vi "CameraOption Disp.vi"() -> ()   [LabVIEW 2015]
uses:
  global.vi
panel:
  in  "タブ制御器":enum32{"I/O", "Partition"}(tab)
  in  "I/O PortSetting":T1={"ExternalOut2"=13, "ExternalIn2"=6, "ExternalOut1"=0, "ExternalIn1"=0, "ExternalOut3"=13, "ExternalOut4"=13, "ExternalIn3"=6} {"ExternalIn3" items=["TRIG POS "=8, "TRIG NEG "=9]; "ExternalOut4" items=["TRIG POS"=5, "TRIG NEG"=6, ""=11, ""=12]; "ExternalOut3" items=["SYNC POS"=1, "SYNC NEG"=2, "EXPOSE POS"=13, "EXPOSE NEG"=14, "REC POS"=3, "REC NEG"=4, "TRIG POS"=5, "TRIG NEG"=6, "READY POS"=7, "READY NEG"=8, "IRIG RESET POS"=9, "IRIG RESET NEG"=10]; "ExternalIn1" items=["OFF"=1, "CAMSYNC_POS"=2, "CAMSYNC_NEG"=3, "OTHERSSYNC_POS"=4, "OTHERSSYNC_NEG"=5]; "ExternalOut1" items=["SYNC POS"=1, "SYNC NEG"=2, "EXPOSE POS"=13, "EXPOSE NEG"=14, "REC POS"=3, "REC NEG"=4, "TRIG POS"=5, "TRIG NEG"=6, "READY POS"=7, "READY NEG"=8, "IRIG RESET POS"=9, "IRIG RESET NEG"=10]; "ExternalIn2" items=["EVENT POS"=6, "EVENT NEG"=7, "TRIG POS "=8, "TRIG NEG "=9, "READY POS "=10, "READY NEG"=11]; "ExternalOut2" items=["SYNC POS"=1, "SYNC NEG"=2, "EXPOSE POS"=13, "EXPOSE NEG"=14, "REC POS"=3, "REC NEG"=4, "TRIG POS"=5, "TRIG NEG"=6, "READY POS"=7, "READY NEG"=8, "IRIG RESET POS"=9, "IRIG RESET NEG"=10]}
  in  "Pre-LUT":T2={"Mode"=0, "Gain"=1.0, "Gamma"=0.01, "Contrast"=0.0, "Brightness"=0.0, "POS/NEG"=enum."POS", "LUT_Cover"=""} {"Brightness" min=-1024.0 max=1023.0 step=1.0 scale=-1024.0..1023.0 scale format="%#.0f"; "Contrast" min=-512.0 max=511.0 step=1.0 scale=-512.0..511.0; "Gamma" min=0.01 max=2.0 step=0.01 scale=0.01..2.0 scale format="%.2f"; "Gain" min=1.0 max=8.0 step=0.1 scale=1.0..8.0 scale format="%.01f"; "Mode" items=["DEF1"=1, "DEF2"=2, "DEF3"=3, "DEF4"=4, "DEF5"=5, "DEF6"=6, "USER1"=11]}
  in  "Color-Temp":T3={"Mode"=0, "Red"=1, "Green"=0, "Blue"=0, "Color_Cover"=""} {"Blue" max=4095 step=1 scale=-1.0..8191.0; "Green" max=4095 step=1 scale=-1.0..8191.0; "Red" max=4095 step=1 scale=-1.0..8191.0; "Mode" items=["5100K"=1, "3100K"=2, "USER1"=3, "USER2"=4]}
  in  "BitSelect":cluster{"BitShift":dbl}={"BitShift"=1.0} {"BitShift" min=0.0 max=4.0 step=1.0 scale=0.0..4.0 scale format="%.01f"}
  in  "PartitionNo":u32 caption="Number" min=1 max=64 step=1
  in  "PartitionList":T4(array[cluster])
  out "BlockInfo":string
  in  "Equalize":bool
  in  "SetpParams":T5
  in  "MCDL":bool caption="AUX IN"
  in  "IRIG":bool caption="AUX IN"
  in  "OK":bool
  in  "Cancel":bool
  # "Upper(default)"
  # "Lower"
  # "bit shift"
  # "Number                  Frame                       Block"
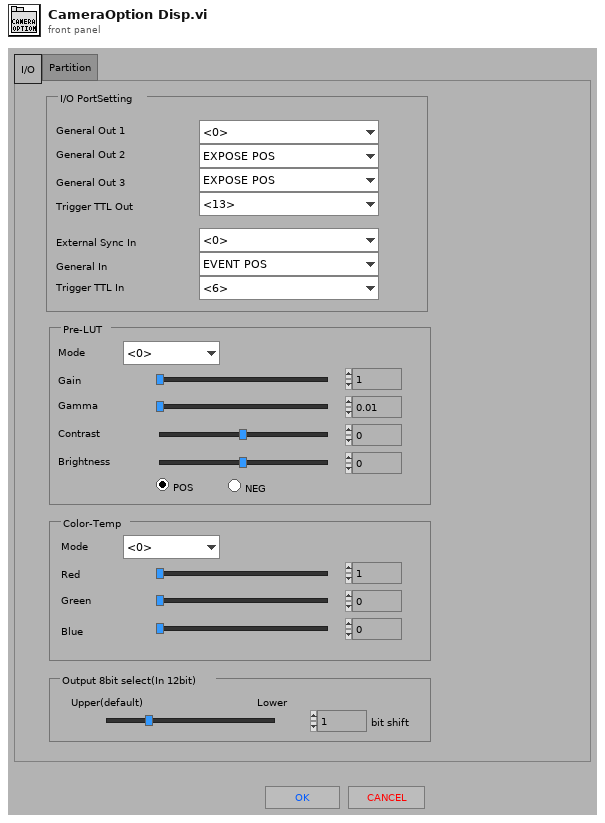
[diagram p1: front panel]
types:
  T1 = cluster{"ExternalOut2":u16, "ExternalIn2":u16, "ExternalOut1":u16, "ExternalIn1":u16, "ExternalOut3":u16, "ExternalOut4":u16, "ExternalIn3":u16}
  T2 = cluster{"Mode":u16, "Gain":dbl, "Gamma":dbl, "Contrast":dbl, "Brightness":dbl, "POS/NEG":enum32{"POS", "NEG"}, "LUT_Cover":string}
  T3 = cluster{"Mode":u32, "Red":u32, "Green":u32, "Blue":u32, "Color_Cover":string}
  T4 = cluster{"Check":bool, "No":string, "Frame":u32, "FrameNo":string, "Block":u32}[]
  T5 = cluster{"m_nBrightnessR":i32, "m_nBrightnessG":i32, "m_nBrightnessB":i32, "m_nContrastR":i32, "m_nContrastG":i32, "m_nContrastB":i32, "m_nGainR":dbl, "m_nGainG":dbl, "m_nGainB":dbl, "m_nGammaR":dbl, "m_nGammaG":dbl, "m_nGammaB":dbl, "m_nPosiNegaR":u8, "m_nPosiNegaG":u8, "m_nPosiNegaB":u8, "m_nFreeMode":u8}
  T6 = cluster{"ReturnValue":u32, "ErrorCode":u32, "error ":errorcluster}
  T7 = cluster{"return type":u32, "pErrorCode":u32, "error ":errorcluster}
  T8 = cluster{"Check":bool, "No":string, "Frame":u32, "FrameNo":string, "Block":u32}
  T9 = cluster{"pCount":u32, "Frames":u32[], "Blocks":u32[], "pNo":u32}
  T10 = cluster{"NewVal":u32, "新規値":u32, "新規値":u32, "新規値":u32}
  T11 = cluster{"Value":u32, "NewVal":u32, "Value":u32, "Value":u32}
  T12 = cluster{"Value":u32, "Value":u32, "NewVal":u32, "Value":u32}
  T13 = cluster{"Value":u32, "Value":u32, "Value":u32, "NewVal":u32}
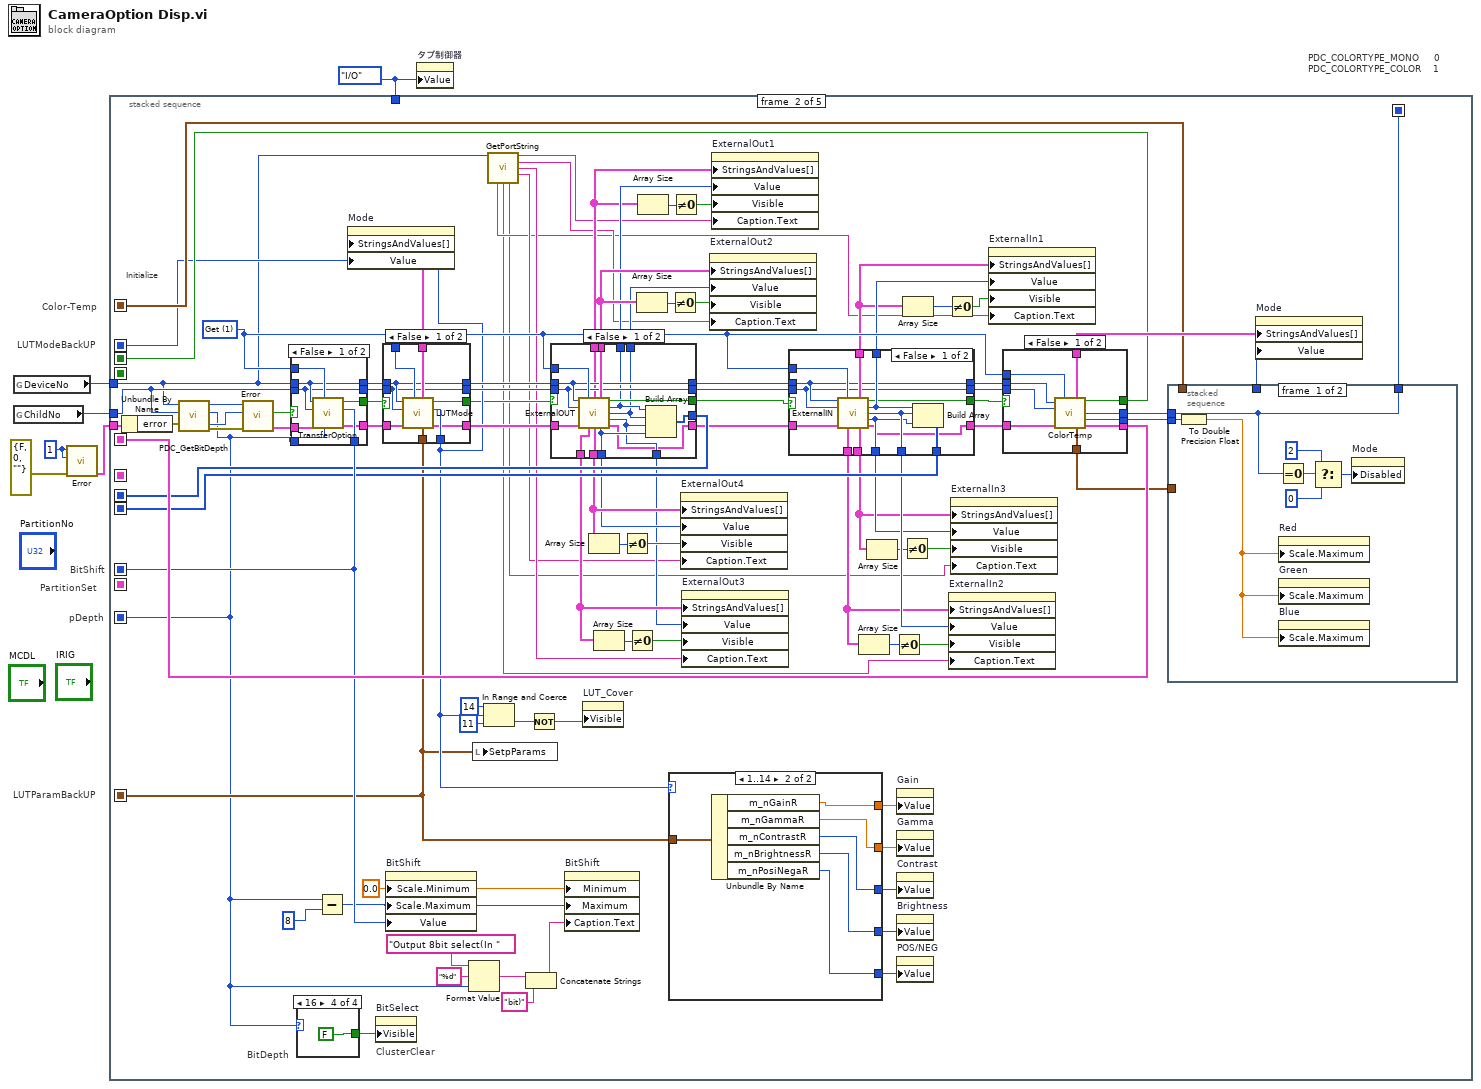
[diagram p0: block diagram]
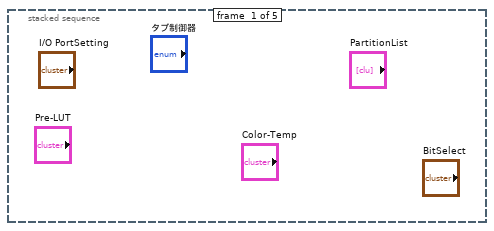
[diagram p2: hidden frame]
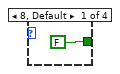
[diagram p3: hidden frame]
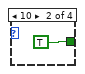
[diagram p4: hidden frame]
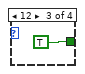
[diagram p5: hidden frame]
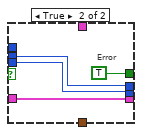
[diagram p6: hidden frame]
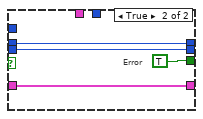
[diagram p7: hidden frame]
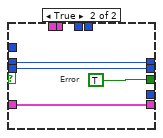
[diagram p8: hidden frame]
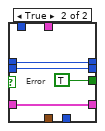
[diagram p9: hidden frame]
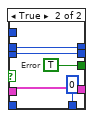
[diagram p10: hidden frame]
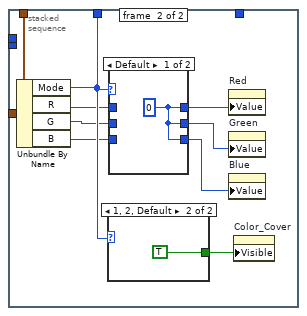
[diagram p11: hidden frame]
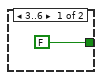
[diagram p12: hidden frame]
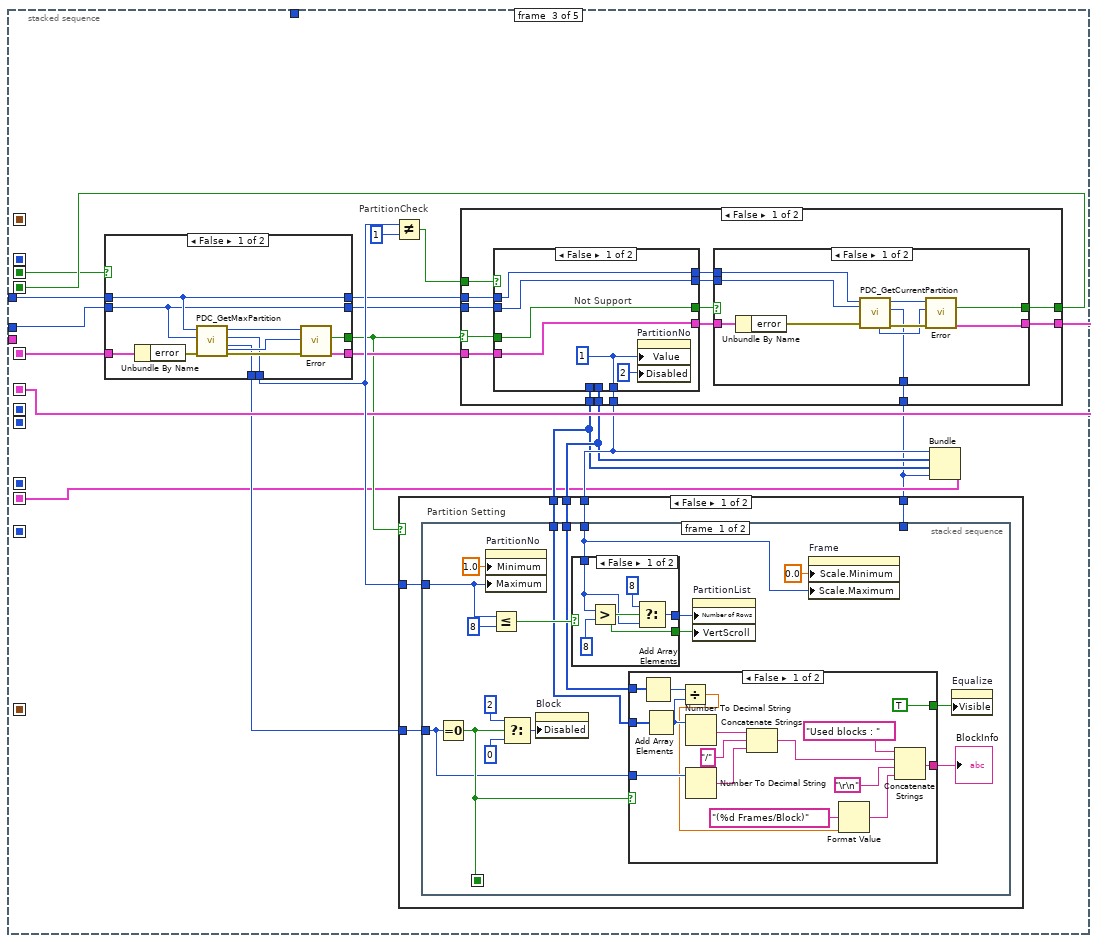
[diagram p15: hidden frame]
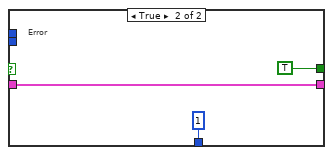
[diagram p16: hidden frame]
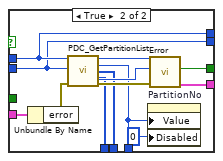
[diagram p17: hidden frame]
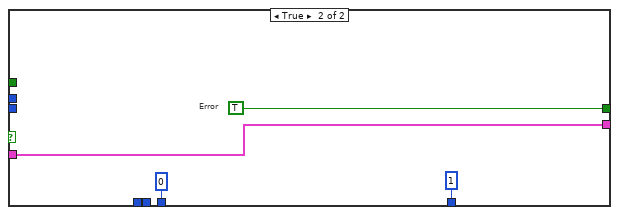
[diagram p18: hidden frame]
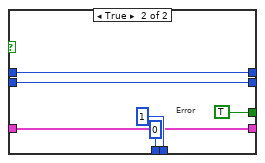
[diagram p19: hidden frame]
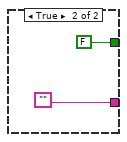
[diagram p20: hidden frame]
diagram:
  w1 = enum32{"I/O", "Partition"}."I/O" ("タブ制御器")
  w4 = u32 1 ("return type")
  # "pDepth"
  # "LUTParamBackUP"
  # "PartitionSet"
  # "PDC_COLORTYPE_MONO\t\t\t\t\t0\nPDC_COLORTYPE_COLOR\t\t\t\t1"
  # "BitShift"
  # "Color-Temp"
  # "LUTModeBackUP"
  n1 = global read "global.vi" "DeviceNo"() -> (w6:u32)
  n2 = global read "global.vi" "ChildNo"() -> (w5:u32)
  n3 = call "Error.vi"("error in (no error)"=errorcluster {"status"=FALSE, "code"=0, "source"=""}, "ErrorCode"=w4, "ReturnValue"=w4) -> ("Error_Out"=w2:T6)  [unwired: 8 out]
  n4 = stacked-sequence {
    seq-local: [_ w51 _ _ _] -> [_ _ _ w382 _]
    seq-local: [_ w96 _ _ _] -> [_ _ w218 _ _]
    seq-local: [_ _ w224 _ _] -> [_ _ _ w381 _]
    seq-local: [_ w85 _ _ _] -> [_ _ _ w379 _]
    seq-local: [_ w84 _ _ _] -> [_ _ _ w380 _]
    seq-local: [_ w77 _ _ _] -> [_ _ _ w378 _]
    seq-local: [_ w76 _ _ _] -> [_ _ _ w377 _]
    seq-local: [_ _ w223 _ _] -> [_ _ _ w376 _]
    seq-local: [_ w54 _ _ _] -> [_ _ w217 _ _]
    seq-local: [_ w52 _ _ _] -> [_ _ _ w375 _]
    seq-local: [_ _ w211 _ _] -> [_ _ _ w373 _]
    seq-local: [_ w48 _ _ _] -> [_ _ _ w374 _]
    seq-local: [_ w39 _ _ _] -> [_ _ _ w372 _]
    tunnel: w6 -> [_ w14 w222 w384 _]
    tunnel: w5 -> [_ w53 w221 w383 _]
    tunnel: w2 -> [_ w83 _ _ _]
    tunnel: w1 -> [_ _ _ _ _]
    frame #0 {
    }
    frame #1 {
      w46 = 0.0 ("スケール.範囲: 最小値")
      w56 = u16 1 items=["Get&Set", "Get", "Set"] ("Mode")
      # "ClusterClear"
      # "BitDepth"
      # "Initialize"
      n5 = Unbundle By Name(w83) -> ("error"=w82:errorcluster)
      n6 = call "PDC_GetBitDepth.vi"("error in (no error)"=w82, "ChildNo"=w53, "DeviceNo"=w14) -> ("error out"=w81:errorcluster, "Depth"=w39:i8, "ReturnValue"=w79:u32, "ErrorCode"=w78:u32)  [unwired: 5 out]
      n7 = call "Error.vi"("error in (no error)"=w81, "ErrorCode"=w78, "ReturnValue"=w79) -> ("Error_Out"=w80:T6, "Error?"=w64:bool)  [unwired: 7 out]
      n8 = case shown="False" w64 {
        tunnel: w56 -> [w176 _]
        tunnel: [w175 u32 0 ("n8BitSel")] -> w84
        tunnel: w80 -> [w174 w179]
        tunnel: w53 -> [w171 w180]
        tunnel: w14 -> [w172 w181]
        tunnel: [w173 w179] -> w75
        tunnel: [w172 w181] -> w66
        tunnel: [w171 w180] -> w65
        tunnel: [w170 TRUE ("Error?")] -> w63
        tunnel: w39 -> [w169 _]
        frame False {
          n9 = call "TransferOption.vi"("Depth"=w169, "Mode"=w176, "Error_In"=w174, "ChildNo"=w171, "DeviceNo"=w172) -> ("Error_Out"=w173:T6, "8BitSel"=w175:u32, "Error?"=w170:bool)  [unwired: 1 in, 2 out]
        }
        frame True {
          # "Error"
        }
      }
      n10 = case shown="16" w39 {
        tunnel: [FALSE TRUE TRUE FALSE] -> w38
        frame 8, Default {
        }
        frame 10 {
        }
        frame 12 {
        }
        frame 16 {
        }
      }
      n11 = Subtract(x=w39, y=i8 8) -> (x-y=w45:i8)
      n12 = property on="BitSelect" class="Clust (strict)"("Visible"=w38) -> ()  [unwired: 2 in, 2 out]
      n13 = case shown="False" w63 {
        tunnel: [w164 _] -> w48
        tunnel: [w163 _] -> w51
        tunnel: w75 -> [w162 w168]
        tunnel: [w161 _] -> w74
        tunnel: [w160 w168] -> w73
        tunnel: w66 -> [w158 w167]
        tunnel: w65 -> [w157 w166]
        tunnel: w56 -> [w159 _]
        tunnel: [w158 w167] -> w62
        tunnel: [w157 w166] -> w60
        tunnel: [w156 TRUE ("Error?")] -> w50
        frame False {
          n14 = call "LUTMode.vi"("Mode"=w159, "Error_In"=w162, "ChildNo"=w157, "DeviceNo"=w158) -> ("Error_Out"=w160:T6, "LUTMode"=w163:u32, "Error?"=w156:bool, "GetpParams"=w164:T5, "LUTModeList"=w161:cluster{string, i32}[])  [unwired: 2 in, 1 out]
        }
        frame True {
          # "Error"
        }
      }
      n15 = property on="Mode" class="Ring (strict)"("StringsAndValues[]"=w74, "Value"=w51) -> ()  [unwired: 2 in, 2 out]
      n16 = property on="BitShift" class="Slide (strict)"("Scale.Minimum"=w46, "Scale.Maximum"=w45, "Value"=w84) -> ()  [unwired: 2 in, 2 out]
      n17 = Format Value(string ("")="Output 8bit select(In ", format string="%d" ("形式文字列"), value (0)=w39) -> (output string=w42:string)
      n18 = local write "SetpParams"(w48) -> ()
      n19 = In Range and Coerce(upper limit=u32 14 ("上限"), x=w51, lower limit=u32 11 ("下限")) -> (In Range?=w88:bool)  [unwired: 1 out]
      n20 = call "GetPortString.vi"("nDeviceNo"=w14) -> ("ExternOut1"=w13:string, "ExternOut2"=w12:string, "ExternOut3"=w11:string, "ExternOut4"=w10:string, "ExternIn1"=w9:string, "ExternIn2"=w8:string, "ExternIn3"=w7:string)  [unwired: 8 out]
      n21 = Concatenate Strings(w42, "bit)") -> (w40:string)
      n22 = Not(x=w88) -> (.not. x?=w87:bool)
      n23 = case shown="False" w50 {
        tunnel: [w137 _] -> w20
        tunnel: [w151 _] -> w77
        tunnel: w73 -> [w150 w152]
        tunnel: [w139 w152] -> w72
        tunnel: [w149 _] -> w70
        tunnel: [w142 _] -> w67
        tunnel: w56 -> [w148 _]
        tunnel: w62 -> [w147 w155]
        tunnel: [w147 w155] -> w61
        tunnel: w60 -> [w146 w154]
        tunnel: [w146 w154] -> w59
        tunnel: [w145 TRUE ("Error?")] -> w49
        tunnel: [w144 _] -> w22
        tunnel: [w143 _] -> w25
        tunnel: [w141 _] -> w19
        tunnel: [w138 _] -> w16
        tunnel: [w140 _] -> w15
        frame False {
          n24 = call "ExternalOUT.vi"("nDeviceNo"=w147, "Mode"=w148, "nChildNo"=w146, "Error_In"=w150) -> ("ExternalOut1ModeList"=w144:cluster{string, i32}[], "ExternalOut2ModeList"=w149:cluster{string, i32}[], "Error?"=w145:bool, "ExternalOut1Mode"=w143:u32, "ExternalOut2Mode"=w142:u32, "ExternalOut3Mode"=w140:u32, "ExternalOut3ModeList"=w138:cluster{string, i32}[], "ExternalOut4ModeList"=w137:cluster{string, i32}[], "ExternalOut4Mode"=w141:u32, "Error_Out"=w139:T7)  [unwired: 1 in, 1 out]
          n25 = Build Array(w143, w142, w140, w141) -> (w151:u32[])
        }
        frame True {
          # "Error"
        }
      }
      n26 = property on="BitShift" class="Slide (strict)"("Minimum"=w46, "Maximum"=w45, "Caption.Text"=w40) -> ()  [unwired: 2 in, 2 out]
      n27 = property on="LUT_Cover" class="Str"("Visible"=w87) -> ()  [unwired: 2 in, 2 out]
      n28 = Array Size(array=w20) -> (size(s)=w91:i32)
      n29 = Array Size(array=w16) -> (size(s)=w18:i32)
      n30 = Not Equal To 0?(x=w91) -> (x != 0?=w21:bool)
      n31 = Not Equal To 0?(x=w18) -> (x != 0?=w17:bool)
      n32 = Array Size(array=w70) -> (size(s)=w69:i32)
      n33 = Array Size(array=w22) -> (size(s)=w24:i32)
      n34 = case shown="1..14" w51 {
        tunnel: [_ w209] -> w101
        tunnel: [_ w208] -> w100
        tunnel: [_ w207] -> w99
        tunnel: [_ w206] -> w98
        tunnel: [_ w205] -> w97
        tunnel: w48 -> [_ w204]
        frame Default {
        }
        frame 1..14 {
          n35 = Unbundle By Name(w204) -> ("m_nGainR"=w209:dbl, "m_nGammaR"=w208:dbl, "m_nContrastR"=w207:i32, "m_nBrightnessR"=w206:i32, "m_nPosiNegaR"=w205:u8)
        }
      }
      n36 = Not Equal To 0?(x=w69) -> (x != 0?=w68:bool)
      n37 = Not Equal To 0?(x=w24) -> (x != 0?=w23:bool)
      n38 = property on="ExternalOut4" class="Ring (strict)"("StringsAndValues[]"=w20, "Value"=w19, "Visible"=w21, "Caption.Text"=w10) -> ()  [unwired: 2 in, 2 out]
      n39 = property on="ExternalOut3" class="Ring (strict)"("StringsAndValues[]"=w16, "Value"=w15, "Visible"=w17, "Caption.Text"=w11) -> ()  [unwired: 2 in, 2 out]
      n40 = property on="ExternalOut2" class="Ring (strict)"("StringsAndValues[]"=w70, "Value"=w67, "Visible"=w68, "Caption.Text"=w12) -> ()  [unwired: 2 in, 2 out]
      n41 = property on="ExternalOut1" class="Ring (strict)"("StringsAndValues[]"=w22, "Value"=w25, "Visible"=w23, "Caption.Text"=w13) -> ()  [unwired: 2 in, 2 out]
      n42 = case shown="False" w49 {
        tunnel: [w132 _] -> w31
        tunnel: [w131 _] -> w76
        tunnel: w72 -> [w130 w136]
        tunnel: [w120 w136] -> w71
        tunnel: [w129 _] -> w33
        tunnel: [w128 _] -> w34
        tunnel: w56 -> [w127 _]
        tunnel: w61 -> [w126 w135]
        tunnel: w59 -> [w125 w134]
        tunnel: [w126 w135] -> w58
        tunnel: [w125 w134] -> w57
        tunnel: [w124 TRUE ("Error?")] -> w55
        tunnel: [w123 _] -> w30
        tunnel: [w122 _] -> w26
        tunnel: [w121 _] -> w29
        frame False {
          n43 = call "ExternalIN.vi"("nDeviceNo"=w126, "Mode"=w127, "nChildNo"=w125, "Error_In"=w130) -> ("ExternalIn1ModeList"=w129:cluster{string, i32}[], "Error?"=w124:bool, "ExternalIn1Mode"=w128:u32, "ExternalIn2Mode"=w132:u32, "ExternalIn3Mode"=w121:u32, "ExternalIn2ModeList"=w123:cluster{string, i32}[], "ExternalIn3ModeList"=w122:cluster{string, i32}[], "Error_Out"=w120:T7)  [unwired: 1 in, 3 out]
          n44 = Build Array(w128, w132, w121) -> (w131:u32[])
        }
        frame True {
          # "Error"
        }
      }
      n45 = Array Size(array=w30) -> (size(s)=w36:i32)
      n46 = Array Size(array=w26) -> (size(s)=w28:i32)
      n47 = Not Equal To 0?(x=w36) -> (x != 0?=w32:bool)
      n48 = property on="Gain" class="Slide (strict)"("Value"=w101) -> ()  [unwired: 2 in, 2 out]
      n49 = property on="Gamma" class="Slide (strict)"("Value"=w100) -> ()  [unwired: 2 in, 2 out]
      n50 = property on="Contrast" class="Slide (strict)"("Value"=w99) -> ()  [unwired: 2 in, 2 out]
      n51 = property on="Brightness" class="Slide (strict)"("Value"=w98) -> ()  [unwired: 2 in, 2 out]
      n52 = property on="POS/NEG" class="RadioBtnsControl (strict)"("Value"=w97) -> ()  [unwired: 2 in, 2 out]
      n53 = Not Equal To 0?(x=w28) -> (x != 0?=w27:bool)
      n54 = Array Size(array=w33) -> (size(s)=w37:i32)
      n55 = Not Equal To 0?(x=w37) -> (x != 0?=w35:bool)
      n56 = property on="ExternalIn2" class="Ring (strict)"("StringsAndValues[]"=w30, "Value"=w31, "Visible"=w32, "Caption.Text"=w8) -> ()  [unwired: 2 in, 2 out]
      n57 = property on="ExternalIn3" class="Ring (strict)"("StringsAndValues[]"=w26, "Value"=w29, "Visible"=w27, "Caption.Text"=w7) -> ()  [unwired: 2 in, 2 out]
      n58 = property on="ExternalIn1" class="Ring (strict)"("StringsAndValues[]"=w33, "Value"=w34, "Visible"=w35, "Caption.Text"=w9) -> ()  [unwired: 2 in, 2 out]
      n59 = case shown="False" w55 {
        tunnel: [w115 w119] -> w96
        tunnel: [w114 _] -> w95
        tunnel: [w113 _] -> w94
        tunnel: [w112 w117] -> w93
        tunnel: [w111 w118] -> w92
        tunnel: w71 -> [w110 w119]
        tunnel: w58 -> [w109 w118]
        tunnel: w57 -> [w108 w117]
        tunnel: w56 -> [w107 _]
        tunnel: [w106 TRUE ("Error?")] -> w54
        frame False {
          n60 = call "ColorTemp.vi"("DeviceNo"=w109, "Mode"=w107, "ChildNo"=w108, "Error_In"=w110) -> ("ColorTempList"=w114:cluster{string, i32}[], "Error?"=w106:bool, "Type"=w111:i8, "Max"=w112:u32, "GetColor"=w113:cluster{"Mode":u32, "R":u32, "G":u32, "B":u32}, "Error_Out"=w115:T6)  [unwired: 1 in, 5 out]
        }
        frame True {
          # "Error"
        }
      }
      n61 = stacked-sequence {
        tunnel: [_ w193] -> w86
        tunnel: w94 -> [_ w189]
        tunnel: w93 -> [w188 _]
        tunnel: w92 -> [w182 _]
        tunnel: [_ w189] -> w85
        tunnel: [w182 _] -> w52
        frame #0 {
          n62 = To Double Precision Float(number=w188) -> (double precision float=w187:dbl)
          n63 = Equal To 0?(x=w182) -> (x = 0?=w186:bool)
          n64 = property on="Red" class="Slide (strict)"("Scale.Maximum"=w187) -> ()  [unwired: 2 in, 2 out]
          n65 = property on="Green" class="Slide (strict)"("Scale.Maximum"=w187) -> ()  [unwired: 2 in, 2 out]
          n66 = property on="Blue" class="Slide (strict)"("Scale.Maximum"=w187) -> ()  [unwired: 2 in, 2 out]
          n67 = Select(t=u8 2, s=w186, f=u8 0) -> (s? t:f=w185:u8)
          n68 = property on="Mode" class="Ring (strict)"("Disabled"=w185) -> ()  [unwired: 2 in, 2 out]
        }
        frame #1 {
          n69 = Unbundle By Name(w189) -> ("Mode"=w193:u32, "R"=w192:u32, "G"=w191:u32, "B"=w190:u32)
          n70 = case shown="1, 2, Default" w193 {
            tunnel: [FALSE ("表示") TRUE ("表示")] -> w194
            frame 3..6 {
            }
            frame 1, 2, Default {
            }
          }
          n71 = case shown="Default" w193 {
            tunnel: [w200 w203] -> w197
            tunnel: [w200 w202] -> w196
            tunnel: [w200 w201] -> w195
            tunnel: w192 -> [_ w203]
            tunnel: w191 -> [_ w202]
            tunnel: w190 -> [_ w201]
            frame Default {
              w200 = u32 0 ("pR")
            }
            frame 1..6 {
            }
          }
          n72 = property on="Red" class="Slide (strict)"("Value"=w197) -> ()  [unwired: 2 in, 2 out]
          n73 = property on="Green" class="Slide (strict)"("Value"=w196) -> ()  [unwired: 2 in, 2 out]
          n74 = property on="Blue" class="Slide (strict)"("Value"=w195) -> ()  [unwired: 2 in, 2 out]
          n75 = property on="Color_Cover" class="Str"("Visible"=w194) -> ()  [unwired: 2 in, 2 out]
        }
      }
      n76 = property on="Mode" class="Ring (strict)"("StringsAndValues[]"=w95, "Value"=w86) -> ()  [unwired: 2 in, 2 out]
    }
    frame #2 {
      # "PartitionCheck"
      n77 = case shown="False" w217 {
        tunnel: [w287 u32 1 ("pCount")] -> w228
        tunnel: [w286 w295] -> w225
        tunnel: [w285 TRUE ("Error?")] -> w216
        tunnel: w222 -> [w284 w293]
        tunnel: w221 -> [w283 w292]
        tunnel: [w284 w293] -> w220
        tunnel: [w283 w292] -> w219
        tunnel: w218 -> [w282 w295]
        tunnel: [w280 u32 0 ("pBlock")] -> w215
        frame False {
          n78 = Unbundle By Name(w282) -> ("error"=w281:errorcluster)
          n79 = call "PDC_GetMaxPartition.vi"("error in (no error)"=w281, "ChildNo"=w283, "DeviceNo"=w284) -> ("error out"=w290:errorcluster, "Block"=w280:u32, "Count"=w287:u32, "ReturnValue"=w289:u32, "ErrorCode"=w288:u32)  [unwired: 4 out]
          n80 = call "Error.vi"("error in (no error)"=w290, "ErrorCode"=w288, "ReturnValue"=w289) -> ("Error_Out"=w286:T6, "Error?"=w285:bool)  [unwired: 7 out]
        }
        frame True {
          # "Error"
        }
      }
      n81 = Not Equal?(x=w228, y=u32 1) -> (x != y?=w226:bool)
      n82 = case shown="False" w216 {
        selector: w216 -> [w239 _]
        tunnel: w226 -> [w243 _]
        tunnel: w225 -> [w242 w278]
        tunnel: [w232 w278] -> w224
        tunnel: [w234 TRUE ("Error?")] -> w223
        tunnel: w220 -> [w241 _]
        tunnel: w219 -> [w240 _]
        tunnel: [w238 u32 0 ("pCount")] -> w214
        tunnel: [w237 _] -> w213
        tunnel: [w236 _] -> w212
        tunnel: [w229 u32 1 ("pNo")] -> w210
        frame False {
          n83 = case shown="False" w243 {
            tunnel: w241 -> [w260 w265]
            tunnel: w240 -> [w259 w264]
            tunnel: w242 -> [w262 w275]
            tunnel: [w262 w270] -> w233
            tunnel: [w261 w269] -> w235
            tunnel: w239 -> [w261 _]
            tunnel: [w257 w268] -> w238
            tunnel: [_ w267] -> w237
            tunnel: [_ w266] -> w236
            tunnel: [w260 w265] -> w231
            tunnel: [w259 w264] -> w230
            frame False {
              w257 = u32 1 ("pCount")
              # "Not Support"
              n84 = property on="PartitionNo" class="DigNum (strict)"("Value"=w257, "Disabled"=u8 2 ("無効")) -> ()  [unwired: 2 in, 2 out]
            }
            frame True {
              n85 = Unbundle By Name(w275) -> ("error"=w274:errorcluster)
              n86 = call "PDC_GetPartitionList.vi"("DeviceNo"=w265, "ChildNo"=w264, "error in (no error)"=w274) -> ("ReturnValue"=w272:u32, "Count"=w268:u32, "Frames"=w267:u32[], "Blocks"=w266:u32[], "ErrorCode"=w271:u32, "error out"=w273:errorcluster)  [unwired: 7 out]
              n87 = property on="PartitionNo" class="DigNum (strict)"("Value"=w268, "Disabled"=u8 0 ("無効")) -> ()  [unwired: 2 in, 2 out]
              n88 = call "Error.vi"("error in (no error)"=w273, "ErrorCode"=w271, "ReturnValue"=w272) -> ("Error_Out"=w270:T6, "Error?"=w269:bool)  [unwired: 7 out]
            }
          }
          n89 = case shown="False" w235 {
            tunnel: [w248 TRUE] -> w234
            tunnel: w233 -> [w253 w256]
            tunnel: [w249 w256] -> w232
            tunnel: w231 -> [w246 _]
            tunnel: w230 -> [w245 _]
            tunnel: [w244 u32 1 ("pNo")] -> w229
            frame False {
              n90 = Unbundle By Name(w253) -> ("error"=w252:errorcluster)
              n91 = call "PDC_GetCurrentPartition.vi"("error in (no error)"=w252, "ChildNo"=w245, "DeviceNo"=w246) -> ("error out"=w250:errorcluster, "No"=w244:u32, "ReturnValue"=w251:u32, "ErrorCode"=w247:u32)  [unwired: 5 out]
              n92 = call "Error.vi"("error in (no error)"=w250, "ErrorCode"=w247, "ReturnValue"=w251) -> ("Error_Out"=w249:T6, "Error?"=w248:bool)  [unwired: 7 out]
            }
            frame True {
              # "Error"
            }
          }
        }
        frame True {
          # "Error"
        }
      }
      n93 = case shown="False" w216 {
        tunnel: w228 -> [w301 _]
        tunnel: w215 -> [w302 _]
        tunnel: w214 -> [w300 _]
        tunnel: w213 -> [w299 _]
        tunnel: w212 -> [w298 _]
        tunnel: w210 -> [w297 _]
        frame False {
          # "Partition Setting"
          n94 = stacked-sequence {
            seq-local: [w308 _] -> [_ w346]
            tunnel: w302 -> [w306 _]
            tunnel: w301 -> [w311 _]
            tunnel: w300 -> [w309 w351]
            tunnel: w299 -> [w304 w350]
            tunnel: w298 -> [w305 w349]
            tunnel: w297 -> [_ w345]
            frame #0 {
              n95 = Equal To 0?(x=w306) -> (x = 0?=w308:bool)
              n96 = property on="PartitionNo" class="DigNum (strict)"("Minimum"=1.0 ("データエントリ制限:最小"), "Maximum"=w311) -> ()  [unwired: 2 in, 2 out]
              n97 = Less Or Equal?(x=w311, y=u32 8) -> (x <= y?=w314:bool)
              n98 = Select(t=u8 2 ("無効"), s=w308, f=u8 0 ("無効")) -> (s? t:f=w316:u8)
              n99 = property on="Block" class="DigNum (strict)"("Disabled"=w316) -> ()  [unwired: 2 in, 2 out]
              n100 = case shown="False" w314 {
                tunnel: [w339 w343] -> w313
                tunnel: [w341 FALSE] -> w312
                tunnel: w309 -> [w338 w343]
                frame False {
                  n101 = Greater?(x=w338, y=u32 8 ("pCount")) -> (0:w341:bool)
                  n102 = Select(t=u32 8 ("pCount"), s=w341, f=w338) -> (s? t:f=w339:u32)
                }
                frame True {
                }
              }
              n103 = case shown="False" w308 {
                tunnel: [w332 ""] -> w307
                tunnel: w306 -> [w326 _]
                tunnel: w305 -> [w325 _]
                tunnel: w304 -> [w324 _]
                tunnel: [TRUE FALSE] -> w303
                frame False {
                  n104 = Add Array Elements(numeric array=w324) -> (sum=w323:u32)
                  n105 = Add Array Elements(numeric array=w325) -> (sum=w322:u32)
                  n106 = Divide(x=w323, y=w322) -> (x/y=w321:dbl)
                  n107 = Number To Decimal String(number=w322) -> (decimal integer string=w330:string)  [unwired: 1 out]
                  n108 = Number To Decimal String(number=w326) -> (decimal integer string=w327:string)  [unwired: 1 out]
                  n109 = Concatenate Strings(w330, "/", w327) -> (w328:string)
                  n110 = Format Value(format string="(%d Frames/Block)" ("形式文字列"), value (0)=w321) -> (output string=w335:string)  [unwired: 1 out]
                  n111 = Concatenate Strings("Used blocks : " ("形式文字列"), w328, "\r\n", w335) -> (w332:string)
                }
                frame True {
                }
              }
              "BlockInfo" <- w307
              n112 = property on="PartitionList" class="Arr (strict)"("Number of Rows"=w313, "VertScroll"=w312) -> ()  [unwired: 2 in, 2 out]
              n113 = property on="Frame" class="Slide (strict)"("Scale.Minimum"=0.0 ("データエントリ制限:最小"), "Scale.Maximum"=w309) -> ()  [unwired: 2 in, 2 out]
              n114 = property on="Equalize" class="Bool"("Visible"=w303) -> ()  [unwired: 2 in, 2 out]
            }
            frame #1 {
              # "<-CurrentPartition"
              n115 = for {
                N: w351 -> [_]
                tunnel: w350 -> [w370]
                tunnel: w349 -> [w369]
                shift-right: [w371] -> w347
                shift-left: T4 [{"Check"=TRUE, "No"="", "Frame"=0, "FrameNo"="", "Block"=0}, {"Check"=FALSE, "No"="", "Frame"=0, "FrameNo"="", "Block"=0}, {"Check"=FALSE, "No"="", "Frame"=0, "FrameNo"="", "Block"=0}, {"Check"=FALSE, "No"="", "Frame"=0, "FrameNo"="", "Block"=0}, {"Check"=FALSE, "No"="", "Frame"=0, "FrameNo"="", "Block"=0}, {"Check"=FALSE, "No"="", "Frame"=0, "FrameNo"="", "Block"=0}, {"Check"=FALSE, "No"="", "Frame"=0, "FrameNo"="", "Block"=0}, {"Check"=FALSE, "No"="", "Frame"=0, "FrameNo"="", "Block"=0}, {"Check"=FALSE, "No"="", "Frame"=0, "FrameNo"="", "Block"=0}, {"Check"=FALSE, "No"="", "Frame"=0, "FrameNo"="", "Block"=0}, {"Check"=FALSE, "No"="", "Frame"=0, "FrameNo"="", "Block"=0}, {"Check"=FALSE, "No"="", "Frame"=0, "FrameNo"="", "Block"=0}, {"Check"=FALSE, "No"="", "Frame"=0, "FrameNo"="", "Block"=0}, {"Check"=FALSE, "No"="", "Frame"=0, "FrameNo"="", "Block"=0}, {"Check"=FALSE, "No"="", "Frame"=0, "FrameNo"="", "Block"=0}, {"Check"=FALSE, "No"="", "Frame"=0, "FrameNo"="", "Block"=0}, {"Check"=FALSE, "No"="", "Frame"=0, "FrameNo"="", "Block"=0}, {"Check"=FALSE, "No"="", "Frame"=0, "FrameNo"="", "Block"=0}, {"Check"=FALSE, "No"="", "Frame"=0, "FrameNo"="", "Block"=0}, {"Check"=FALSE, "No"="", "Frame"=0, "FrameNo"="", "Block"=0}, {"Check"=FALSE, "No"="", "Frame"=0, "FrameNo"="", "Block"=0}, {"Check"=FALSE, "No"="", "Frame"=0, "FrameNo"="", "Block"=0}, {"Check"=FALSE, "No"="", "Frame"=0, "FrameNo"="", "Block"=0}, {"Check"=FALSE, "No"="", "Frame"=0, "FrameNo"="", "Block"=0}, {"Check"=FALSE, "No"="", "Frame"=0, "FrameNo"="", "Block"=0}, {"Check"=FALSE, "No"="", "Frame"=0, "FrameNo"="", "Block"=0}, {"Check"=FALSE, "No"="", "Frame"=0, "FrameNo"="", "Block"=0}, {"Check"=FALSE, "No"="", "Frame"=0, "FrameNo"="", "Block"=0}, {"Check"=FALSE, "No"="", "Frame"=0, "FrameNo"="", "Block"=0}, {"Check"=FALSE, "No"="", "Frame"=0, "FrameNo"="", "Block"=0}, {"Check"=FALSE, "No"="", "Frame"=0, "FrameNo"="", "Block"=0}, {"Check"=FALSE, "No"="", "Frame"=0, "FrameNo"="", "Block"=0}, {"Check"=FALSE, "No"="", "Frame"=0, "FrameNo"="", "Block"=0}, {"Check"=FALSE, "No"="", "Frame"=0, "FrameNo"="", "Block"=0}, {"Check"=FALSE, "No"="", "Frame"=0, "FrameNo"="", "Block"=0}, {"Check"=FALSE, "No"="", "Frame"=0, "FrameNo"="", "Block"=0}, {"Check"=FALSE, "No"="", "Frame"=0, "FrameNo"="", "Block"=0}, {"Check"=FALSE, "No"="", "Frame"=0, "FrameNo"="", "Block"=0}, {"Check"=FALSE, "No"="", "Frame"=0, "FrameNo"="", "Block"=0}, {"Check"=FALSE, "No"="", "Frame"=0, "FrameNo"="", "Block"=0}, {"Check"=FALSE, "No"="", "Frame"=0, "FrameNo"="", "Block"=0}, {"Check"=FALSE, "No"="", "Frame"=0, "FrameNo"="", "Block"=0}, {"Check"=FALSE, "No"="", "Frame"=0, "FrameNo"="", "Block"=0}, {"Check"=FALSE, "No"="", "Frame"=0, "FrameNo"="", "Block"=0}, {"Check"=FALSE, "No"="", "Frame"=0, "FrameNo"="", "Block"=0}, {"Check"=FALSE, "No"="", "Frame"=0, "FrameNo"="", "Block"=0}, {"Check"=FALSE, "No"="", "Frame"=0, "FrameNo"="", "Block"=0}, {"Check"=FALSE, "No"="", "Frame"=0, "FrameNo"="", "Block"=0}, {"Check"=FALSE, "No"="", "Frame"=0, "FrameNo"="", "Block"=0}, {"Check"=FALSE, "No"="", "Frame"=0, "FrameNo"="", "Block"=0}, {"Check"=FALSE, "No"="", "Frame"=0, "FrameNo"="", "Block"=0}, {"Check"=FALSE, "No"="", "Frame"=0, "FrameNo"="", "Block"=0}, {"Check"=FALSE, "No"="", "Frame"=0, "FrameNo"="", "Block"=0}, {"Check"=FALSE, "No"="", "Frame"=0, "FrameNo"="", "Block"=0}, {"Check"=FALSE, "No"="", "Frame"=0, "FrameNo"="", "Block"=0}, {"Check"=FALSE, "No"="", "Frame"=0, "FrameNo"="", "Block"=0}, {"Check"=FALSE, "No"="", "Frame"=0, "FrameNo"="", "Block"=0}, {"Check"=FALSE, "No"="", "Frame"=0, "FrameNo"="", "Block"=0}, {"Check"=FALSE, "No"="", "Frame"=0, "FrameNo"="", "Block"=0}, {"Check"=FALSE, "No"="", "Frame"=0, "FrameNo"="", "Block"=0}, {"Check"=FALSE, "No"="", "Frame"=0, "FrameNo"="", "Block"=0}, {"Check"=FALSE, "No"="", "Frame"=0, "FrameNo"="", "Block"=0}, {"Check"=FALSE, "No"="", "Frame"=0, "FrameNo"="", "Block"=0}, {"Check"=FALSE, "No"="", "Frame"=0, "FrameNo"="", "Block"=0}] ("PartitionList") -> [w368]
                tunnel: w346 -> [w359]
                tunnel: w345 -> [w354]
                i -> [w355]
                n116 = Increment(x=w355) -> (x+1=w366:i32)
                n117 = Increment(x=w355) -> (x+1=w353:i32)
                n118 = Index Array(array=w370, index=w355) -> (element=w362:u32)
                n119 = Index Array(array=w369, index=w355) -> (element=w358:u32)
                n120 = Equal?(x=w353, y=w354) -> (x = y?=w352:bool)
                n121 = Format Value(format string="%03d" ("形式文字列"), value (0)=w366) -> (output string=w364:string)  [unwired: 1 out]
                n122 = Index Array(array=w368, index=w355) -> (element=w367:T8)
                n123 = Select(t=u32 1, s=w359, f=w358) -> (s? t:f=w356:u32)
                n124 = Format Value(format string="%dFrame" ("形式文字列"), value (0)=w362) -> (output string=w361:string)  [unwired: 1 out]
                n125 = Bundle By Name(cluster=w367, "No"=w364, "FrameNo"=w361, "Block"=w356, "Frame"=w356, "Check"=w352) -> (w360:T8)
                n126 = Replace Array Subset(array=w368, new element=w360, index=w355) -> (w371:T4)
              }
              n127 = local write "PartitionList"(w347) -> ()
            }
          }
        }
        frame True {
        }
      }
      n128 = Bundle("pCount"=w214, "Frames"=w213, "Blocks"=w212, "pNo"=w210) -> (w211:T9)  [unwired: 1 out]
    }
    frame #3 {
      n129 = while {
        tunnel: w384 -> [w398]
        tunnel: w383 -> [w399]
        shift-right: [w396] -> _
        shift-left: w381 -> [w397]
        shift-right: [w395] -> _
        shift-left: w376 -> [w394]
        tunnel: w382 -> [w393]
        tunnel: w380 -> [w392]
        tunnel: w379 -> [w391]
        tunnel: w378 -> [w390]
        tunnel: w377 -> [w389]
        tunnel: w375 -> [w388]
        tunnel: w374 -> [w387]
        tunnel: w373 -> [w386]
        tunnel: w372 -> [w385]
        stop <- w400 stop-if-true
        n130 = event shown="[10] \"I/O PortSetting.ExternalOut1\", \"I/O PortSetting.ExternalOut2\", \"I/O PortSetting.ExternalOut3\", \"I/O PortSetting.ExternalOut4\": Value Change" {
          selector: _ -> [_ _ _ _ _ _ _ _ _ _ _ _ _ _]
          dyn-events: _ -> [_ _ _ _ _ _ _ _ _ _ _ _ _ _]
          timeout: 50 -> [_ _ _ _ _ _ _ _ _ _ _ _ _ _]
          tunnel: [w402 TRUE TRUE FALSE FALSE FALSE FALSE FALSE FALSE FALSE FALSE FALSE FALSE FALSE] -> w400
          tunnel: w399 -> [_ _ w482 w611 w659 w706 w752 w798 w844 w885 w908 w943 w986 w1155]
          tunnel: w398 -> [_ _ w483 w612 w660 w707 w753 w799 w845 w884 w909 w944 w987 w1156]
          tunnel: w397 -> [w404 w431 w468 w616 w664 w702 w748 w794 w840 w890 w910 w945 w1000 w1160]
          tunnel: [w403 w431 w453 w609 w657 w708 w754 w800 w846 w889 w906 w942 w995 w1158] -> w396
          tunnel: [w405 w430 w454 w610 w658 w709 w755 w801 w847 w888 w907 w941 w996 w1157] -> w395
          tunnel: w394 -> [w406 w430 _ _ _ _ _ _ _ _ _ _ _ w1159]
          tunnel: w393 -> [_ _ w467 _ _ _ _ _ _ _ _ _ _ _]
          tunnel: w392 -> [_ _ w513 _ _ _ _ _ _ _ _ _ _ _]
          tunnel: w391 -> [_ _ w512 _ _ _ _ _ _ _ _ _ _ _]
          tunnel: w390 -> [_ _ w493 _ _ _ _ _ _ _ _ _ _ _]
          tunnel: w389 -> [_ _ w486 _ _ _ _ _ _ _ _ _ _ _]
          tunnel: w388 -> [_ _ w471 _ _ _ _ _ _ _ _ _ _ _]
          tunnel: [_ "OK" _ _ _ _ _ _ _ _ _ _ _ _] -> _
          tunnel: w387 -> [_ _ w465 _ _ _ _ _ _ _ _ _ _ _]
          tunnel: w386 -> [_ _ w435 _ _ _ _ _ _ _ _ _ _ _]
          tunnel: [_ _ _ _ _ _ _ _ _ _ _ _ w972 _] -> _
          tunnel: [_ _ _ _ _ _ _ _ _ _ _ _ "Equalize" _] -> _
          tunnel: w385 -> [_ _ w451 _ _ _ _ _ _ w881 _ _ _ _]
          event Timeout {
            n131 = event-data() -> ()  [unwired: 3 out]
            n132 = case shown="True" w406 {
              selector: w406 -> [w409 _]
              tunnel: [w409 FALSE] -> w405
              tunnel: w404 -> [w408 w412]
              tunnel: [w408 T7 {"return type"=1, "pErrorCode"=1, "error "={"status"=FALSE, "code"=0, "source"=""}} ("Error_Out")] -> w403
              tunnel: [FALSE TRUE] -> w402
              frame False {
              }
              frame True {
                w428 = "\r\n"
                n133 = Unbundle By Name(w412) -> ("error"=w413:errorcluster, "error.source"=w416:string, "error.code"=w417:i32, "ReturnValue"=w420:u32, "ErrorCode"=w421:u32)
                n134 = Number To Decimal String(number=w417) -> (decimal integer string=w419:string)  [unwired: 1 out]
                n135 = Number To Decimal String(number=w420) -> (decimal integer string=w423:string)  [unwired: 1 out]
                n136 = Number To Decimal String(number=w421) -> (decimal integer string=w425:string)  [unwired: 1 out]
                n137 = call <vilib>:"Clear Errors.vi"("error in (no error)"=w413) -> ("error out"=w414:errorcluster)  [unwired: 1 in, 5 out]
                n138 = Concatenate Strings("<<Error !!>>", w428, w428, w428, "Source=", w416, w428, "LabError=", w419, w428, "ReturnType=", w423, w428, "ErrorCode=", w425) -> (w426:string)
                n139 = call "メッセージ表示"("error in (no error)"=w414, "Message"=w426) -> ()  [unwired: 1 in, 9 out]
              }
            }
          }
          event "OK": Value Change {
            n140 = event-data() -> ()  [unwired: 7 out]
            n141 = case shown="False" w430 {
              frame False {
                n142 = global write "global.vi" "OptionOK"(TRUE ("OptionOK")) -> ()
              }
              frame True {
              }
            }
          }
          event "Cancel": Value Change {
            w466 = u16 2 items=["Get&Set", "Get", "Set"] ("Mode")
            # "Backup"
            n143 = event-data() -> ()  [unwired: 2 out]
            n144 = call "LUTMode.vi"("SetpParams"=w465, "Mode"=w466, "Error_In"=w468, "NewLUTMode"=w467, "ChildNo"=w482, "DeviceNo"=w483) -> ("Error_Out"=w469:T6, "Error?"=w470:bool)  [unwired: 4 out]
            n145 = Not Equal To 0?(x=w471) -> (x != 0?=w472:bool)
            n146 = case shown="True" w472 {
              tunnel: w469 -> [w546 w556]
              tunnel: [w546 w555] -> w514
              tunnel: w512 -> [_ w554]
              tunnel: w483 -> [w543 w553]
              tunnel: w482 -> [w544 w552]
              tunnel: w466 -> [_ w551]
              tunnel: w470 -> [w545 w550]
              tunnel: [w543 w549] -> w481
              tunnel: [w544 w548] -> w480
              tunnel: [w545 w547] -> w479
              frame False {
                # "ColorType=MONO"
              }
              frame True {
                n147 = case shown="False" w550 {
                  tunnel: w556 -> [w563 w565]
                  tunnel: [w562 w565] -> w555
                  tunnel: w554 -> [w561 _]
                  tunnel: w553 -> [w559 w567]
                  tunnel: w552 -> [w558 w566]
                  tunnel: w551 -> [w560 _]
                  tunnel: [w559 w567] -> w549
                  tunnel: [w558 w566] -> w548
                  tunnel: [w557 TRUE ("Error?")] -> w547
                  frame False {
                    n148 = call "ColorTemp.vi"("DeviceNo"=w559, "Mode"=w560, "ChildNo"=w558, "Error_In"=w563, "SetColor"=w561) -> ("Error?"=w557:bool, "Error_Out"=w562:T6)  [unwired: 9 out]
                  }
                  frame True {
                    # "Error"
                  }
                }
              }
            }
            n149 = Index Array(array=w493, index #1=0 ("指標"), index #2=1 ("指標"), index #3=2 ("指標"), index #4=3 ("指標")) -> (element #1=w490:u32, element #2=w489:u32, element #3=w439:u32, element #4=w438:u32)
            n150 = Index Array(array=w486, index #1=0 ("指標"), index #2=1 ("指標"), index #3=2 ("指標")) -> (element #1=w485:u32, element #2=w484:u32, element #3=w448:u32)
            n151 = case shown="False" w479 {
              tunnel: w514 -> [w597 w601]
              tunnel: w513 -> [w596 _]
              tunnel: [w595 w601] -> w494
              tunnel: w466 -> [w594 _]
              tunnel: w481 -> [w592 w599]
              tunnel: w480 -> [w591 w598]
              tunnel: [w593 TRUE ("Error?")] -> w476
              tunnel: [w592 w599] -> w478
              tunnel: [w591 w598] -> w477
              tunnel: w451 -> [w590 _]
              frame False {
                n152 = call "TransferOption.vi"("Depth"=w590, "Mode"=w594, "Error_In"=w597, "Newn8BitSel"=w596, "ChildNo"=w591, "DeviceNo"=w592) -> ("Error_Out"=w595:T6, "Error?"=w593:bool)  [unwired: 3 out]
              }
              frame True {
                # "Error"
              }
            }
            n153 = property on="ExternalOut1" class="Ring (strict)"() -> ("Visible"=w510:bool)  [unwired: 2 in, 2 out]
            n154 = property on="ExternalOut4" class="Ring (strict)"() -> ("Visible"=w441:bool)  [unwired: 2 in, 2 out]
            n155 = property on="ExternalOut2" class="Ring (strict)"() -> ("Visible"=w509:bool)  [unwired: 2 in, 2 out]
            n156 = property on="ExternalOut3" class="Ring (strict)"() -> ("Visible"=w443:bool)  [unwired: 2 in, 2 out]
            n157 = Select(t=w489, s=w509, f=u32 0) -> (s? t:f=w505:u32)
            n158 = Select(t=w439, s=w443, f=u32 0) -> (s? t:f=w437:u32)
            n159 = Select(t=w438, s=w441, f=u32 0) -> (s? t:f=w436:u32)
            n160 = Select(t=w490, s=w510, f=u32 0) -> (s? t:f=w506:u32)
            n161 = Build Array(w506, w505, w437, w436) -> (w504:u32[])
            n162 = To Unsigned Long Integer(number=w504) -> (unsigned 32bit integer=w503:u32[])
            n163 = case shown="False" w476 {
              tunnel: [w585 w589] -> w511
              tunnel: w503 -> [w584 _]
              tunnel: w494 -> [w583 w589]
              tunnel: w466 -> [w582 _]
              tunnel: w478 -> [w580 w587]
              tunnel: w477 -> [w579 w586]
              tunnel: [w581 TRUE ("Error?")] -> w473
              tunnel: [w580 w587] -> w475
              tunnel: [w579 w586] -> w474
              frame False {
                n164 = call "ExternalOUT.vi"("nDeviceNo"=w580, "Mode"=w582, "nChildNo"=w579, "NewExternalOutMode"=w584, "Error_In"=w583) -> ("Error?"=w581:bool, "Error_Out"=w585:T7)  [unwired: 9 out]
              }
              frame True {
                # "Error"
              }
            }
            n165 = property on="ExternalIn1" class="Ring (strict)"() -> ("Visible"=w496:bool)  [unwired: 2 in, 2 out]
            n166 = property on="ExternalIn3" class="Ring (strict)"() -> ("Visible"=w449:bool)  [unwired: 2 in, 2 out]
            n167 = property on="ExternalIn2" class="Ring (strict)"() -> ("Visible"=w495:bool)  [unwired: 2 in, 2 out]
            n168 = Select(t=w484, s=w495, f=u16 0) -> (s? t:f=w501:u32)
            n169 = Unbundle(w435) -> ("pCount"=w460:u32, "Blocks"=w459:u32[], "pNo"=w452:u32)  [unwired: 1 out]
            n170 = Select(t=w448, s=w449, f=u16 0) -> (s? t:f=w447:u32)
            n171 = Select(t=w485, s=w496, f=u16 0) -> (s? t:f=w500:u32)
            n172 = Build Array(w500, w501, w447) -> (w502:u32[])
            n173 = To Unsigned Long Integer(number=w502) -> (unsigned 32bit integer=w497:u32[])
            n174 = case shown="False" w473 {
              tunnel: w511 -> [w574 w578]
              tunnel: w497 -> [w573 _]
              tunnel: [w572 w578] -> w463
              tunnel: [w571 TRUE ("Error?")] -> w464
              tunnel: w466 -> [w570 _]
              tunnel: w475 -> [w569 w576]
              tunnel: w474 -> [w568 w575]
              tunnel: [w569 w576] -> w462
              tunnel: [w568 w575] -> w461
              frame False {
                n175 = call "ExternalIN.vi"("nDeviceNo"=w569, "Mode"=w570, "nChildNo"=w568, "NewExternalInMode"=w573, "Error_In"=w574) -> ("Error?"=w571:bool, "Error_Out"=w572:T7)  [unwired: 9 out]
              }
              frame True {
                # "Error"
              }
            }
            n176 = case shown="False" w464 {
              tunnel: w463 -> [w538 w541]
              tunnel: w462 -> [w529 w540]
              tunnel: w461 -> [w528 w539]
              tunnel: w460 -> [w536 _]
              tunnel: w459 -> [w535 _]
              tunnel: [w531 TRUE ("Error?")] -> w458
              tunnel: [w530 w541] -> w457
              tunnel: [w529 w540] -> w456
              tunnel: [w528 w539] -> w455
              frame False {
                n177 = Unbundle By Name(w538) -> ("error"=w537:errorcluster)
                n178 = call "PDC_SetPartitionList.vi"("Blocks"=w535, "error in (no error)"=w537, "Count"=w536, "ChildNo"=w528, "DeviceNo"=w529) -> ("error out"=w533:errorcluster, "ReturnValue"=w534:u32, "ErrorCode"=w532:u32)  [unwired: 4 out]
                n179 = call "Error.vi"("error in (no error)"=w533, "ErrorCode"=w532, "ReturnValue"=w534) -> ("Error_Out"=w530:T6, "Error?"=w531:bool)  [unwired: 7 out]
              }
              frame True {
                # "Error"
              }
            }
            n180 = case shown="False" w458 {
              tunnel: w457 -> [w525 w526]
              tunnel: w456 -> [w523 _]
              tunnel: w455 -> [w522 _]
              tunnel: [w518 TRUE ("Error?")] -> w454
              tunnel: [w517 w526] -> w453
              tunnel: w452 -> [w516 _]
              frame False {
                n181 = Unbundle By Name(w525) -> ("error"=w524:errorcluster)
                n182 = call "PDC_SetCurrentPartition.vi"("error in (no error)"=w524, "No"=w516, "ChildNo"=w522, "DeviceNo"=w523) -> ("error out"=w520:errorcluster, "ReturnValue"=w521:u32, "ErrorCode"=w519:u32)  [unwired: 5 out]
                n183 = call "Error.vi"("error in (no error)"=w520, "ErrorCode"=w519, "ReturnValue"=w521) -> ("Error_Out"=w517:T6, "Error?"=w518:bool)  [unwired: 7 out]
              }
              frame True {
                # "Error"
              }
            }
            n184 = case shown="False" w454 {
              frame False {
                n185 = global write "global.vi" "OptionOK"(TRUE ("OptionOK")) -> ()
              }
              frame True {
              }
            }
          }
          event "Pre-LUT.Mode": Value Change {
            w615 = u16 2 items=["Get&Set", "Get", "Set"] ("Mode")
            n186 = event-data() -> ("NewVal"=w605:u16)  [unwired: 1 out]
            n187 = In Range and Coerce(upper limit=u32 14 ("上限"), x=w605, lower limit=u32 11 ("下限")) -> (In Range?=w606:bool)  [unwired: 1 out]
            n188 = local read "SetpParams"() -> (w603:T5)
            n189 = Not(x=w606) -> (.not. x?=w604:bool)
            n190 = call "LUTMode.vi"("SetpParams"=w603, "Mode"=w615, "Error_In"=w616, "NewLUTMode"=w605, "ChildNo"=w611, "DeviceNo"=w612) -> ("Error_Out"=w613:T6, "Error?"=w614:bool)  [unwired: 4 out]
            n191 = property on="LUT_Cover" class="Str"("Visible"=w604) -> ()  [unwired: 2 in, 2 out]
            n192 = case shown="False" w614 {
              tunnel: w613 -> [w624 w647]
              tunnel: w612 -> [w623 _]
              tunnel: w611 -> [w622 _]
              tunnel: [w620 TRUE ("Error?")] -> w610
              tunnel: [w621 w647] -> w609
              frame False {
                n193 = flat-sequence {
                  tunnel: w624 -> [w632]
                  tunnel: w623 -> [w631]
                  tunnel: w622 -> [w630]
                  tunnel: [w628] -> w619
                  tunnel: [w626] -> w618
                  tunnel: [w644] -> w620
                  tunnel: [w645] -> w621
                  tunnel: w619 -> [w645]
                  tunnel: w618 -> [w644]
                  frame #0 {
                    w629 = u16 1 items=["Get&Set", "Get", "Set"] ("Mode")
                    n194 = call "LUTMode.vi"("Mode"=w629, "Error_In"=w632, "ChildNo"=w630, "DeviceNo"=w631) -> ("Error_Out"=w628:T6, "LUTMode"=w627:u32, "Error?"=w626:bool, "GetpParams"=w625:T5)  [unwired: 2 in, 2 out]
                    n195 = case shown="1..14" w627 {
                      tunnel: [_ w643] -> w637
                      tunnel: [_ w642] -> w636
                      tunnel: [_ w641] -> w635
                      tunnel: [_ w640] -> w634
                      tunnel: [_ w639] -> w633
                      tunnel: w625 -> [_ w638]
                      frame Default {
                      }
                      frame 1..14 {
                        n196 = Unbundle By Name(w638) -> ("m_nGainR"=w643:dbl, "m_nGammaR"=w642:dbl, "m_nContrastR"=w641:i32, "m_nBrightnessR"=w640:i32, "m_nPosiNegaR"=w639:u8)
                        n197 = local write "SetpParams"(w638) -> ()
                      }
                    }
                    n198 = property on="Gain" class="Slide (strict)"("Value"=w637) -> ()  [unwired: 2 in, 2 out]
                    n199 = property on="Gamma" class="Slide (strict)"("Value"=w636) -> ()  [unwired: 2 in, 2 out]
                    n200 = property on="Contrast" class="Slide (strict)"("Value"=w635) -> ()  [unwired: 2 in, 2 out]
                    n201 = property on="Brightness" class="Slide (strict)"("Value"=w634) -> ()  [unwired: 2 in, 2 out]
                    n202 = property on="POS/NEG" class="RadioBtnsControl (strict)"("Value"=w633) -> ()  [unwired: 2 in, 2 out]
                  }
                  frame #1 {
                    n203 = case shown="False" w644 {
                      frame False {
                        n204 = global write "global.vi" "OptionOK"(TRUE ("OptionOK")) -> ()
                      }
                      frame True {
                      }
                    }
                  }
                }
              }
              frame True {
              }
            }
          }
          event "Pre-LUT.Gain", "Pre-LUT.Gamma", "Pre-LUT.Contrast", "Pre-LUT.Brightness", "Pre-LUT.POS/NEG": Value Change {
            w663 = u16 2 items=["Get&Set", "Get", "Set"] ("Mode")
            n205 = event-data() -> ()  [unwired: 2 out]
            n206 = property on="Gain" class="Slide (strict)"() -> ("Value"=w653:dbl)  [unwired: 2 in, 2 out]
            n207 = property on="Gamma" class="Slide (strict)"() -> ("Value"=w652:dbl)  [unwired: 2 in, 2 out]
            n208 = property on="Contrast" class="Slide (strict)"() -> ("Value"=w651:dbl)  [unwired: 2 in, 2 out]
            n209 = property on="Brightness" class="Slide (strict)"() -> ("Value"=w650:dbl)  [unwired: 2 in, 2 out]
            n210 = property on="POS/NEG" class="RadioBtnsControl (strict)"() -> ("Value"=w649:enum32{"POS", "NEG"})  [unwired: 2 in, 2 out]
            n211 = property on="Mode" class="Ring (strict)"() -> ("Value"=w656:u16)  [unwired: 2 in, 2 out]
            n212 = Bundle By Name(cluster="SetpParams", "m_nGainR"=w653, "m_nGammaR"=w652, "m_nContrastR"=w651, "m_nBrightnessR"=w650, "m_nPosiNegaR"=w649) -> (w654:T5)
            n213 = call "LUTMode.vi"("SetpParams"=w654, "Mode"=w663, "Error_In"=w664, "NewLUTMode"=w656, "ChildNo"=w659, "DeviceNo"=w660) -> ("Error_Out"=w661:T6, "Error?"=w662:bool)  [unwired: 4 out]
            n214 = case shown="False" w662 {
              tunnel: w661 -> [w673 w697]
              tunnel: w660 -> [w672 _]
              tunnel: w659 -> [w671 _]
              tunnel: [w670 TRUE ("Error?")] -> w658
              tunnel: [w669 w697] -> w657
              tunnel: w656 -> [w668 _]
              frame False {
                n215 = flat-sequence {
                  tunnel: w673 -> [w682]
                  tunnel: w672 -> [w681]
                  tunnel: w671 -> [w680]
                  tunnel: w668 -> [w674]
                  tunnel: [w678] -> w667
                  tunnel: [w677] -> w666
                  tunnel: [w695] -> w669
                  tunnel: [w694] -> w670
                  tunnel: w667 -> [w694]
                  tunnel: w666 -> [w695]
                  frame #0 {
                    w679 = u16 1 items=["Get&Set", "Get", "Set"] ("Mode")
                    n216 = call "LUTMode.vi"("Mode"=w679, "Error_In"=w682, "NewLUTMode"=w674, "ChildNo"=w680, "DeviceNo"=w681) -> ("Error_Out"=w677:T6, "LUTMode"=w675:u32, "Error?"=w678:bool, "GetpParams"=w676:T5)  [unwired: 1 in, 2 out]
                    n217 = case shown="1..14" w675 {
                      tunnel: [_ w693] -> w687
                      tunnel: [_ w692] -> w686
                      tunnel: [_ w691] -> w685
                      tunnel: [_ w690] -> w684
                      tunnel: [_ w689] -> w683
                      tunnel: w676 -> [_ w688]
                      frame Default {
                      }
                      frame 1..14 {
                        n218 = Unbundle By Name(w688) -> ("m_nGainR"=w693:dbl, "m_nGammaR"=w692:dbl, "m_nContrastR"=w691:i32, "m_nBrightnessR"=w690:i32, "m_nPosiNegaR"=w689:u8)
                        n219 = local write "SetpParams"(w688) -> ()
                      }
                    }
                    n220 = property on="Gain" class="Slide (strict)"("Value"=w687) -> ()  [unwired: 2 in, 2 out]
                    n221 = property on="Gamma" class="Slide (strict)"("Value"=w686) -> ()  [unwired: 2 in, 2 out]
                    n222 = property on="Contrast" class="Slide (strict)"("Value"=w685) -> ()  [unwired: 2 in, 2 out]
                    n223 = property on="Brightness" class="Slide (strict)"("Value"=w684) -> ()  [unwired: 2 in, 2 out]
                    n224 = property on="POS/NEG" class="RadioBtnsControl (strict)"("Value"=w683) -> ()  [unwired: 2 in, 2 out]
                  }
                  frame #1 {
                    n225 = case shown="False" w694 {
                      frame False {
                        n226 = global write "global.vi" "OptionOK"(TRUE ("OptionOK")) -> ()
                      }
                      frame True {
                      }
                    }
                  }
                }
              }
              frame True {
              }
            }
          }
          event "Color-Temp.Mode": Value Change {
            w705 = u16 2 items=["Get&Set", "Get", "Set"] ("Mode")
            w699 = u32 4294967295 ("新規値")
            n227 = event-data() -> ("NewVal"=w701:u32)  [unwired: 1 out]
            n228 = Bundle("NewVal"=w701, "新規値"=w699, "新規値"=w699, "新規値"=w699) -> (w700:T10)  [unwired: 1 out]
            n229 = call "ColorTemp.vi"("DeviceNo"=w707, "Mode"=w705, "ChildNo"=w706, "Error_In"=w702, "SetColor"=w700) -> ("Error?"=w704:bool, "Error_Out"=w703:T6)  [unwired: 9 out]
            n230 = case shown="False" w704 {
              tunnel: w703 -> [w713 w741]
              tunnel: w707 -> [w716 _]
              tunnel: w706 -> [w715 _]
              tunnel: [w717 TRUE ("Error?")] -> w709
              tunnel: [w714 w741] -> w708
              frame False {
                n231 = flat-sequence {
                  tunnel: w716 -> [w730]
                  tunnel: w715 -> [w729]
                  tunnel: w713 -> [w727]
                  tunnel: [w731] -> w712
                  tunnel: [w728] -> w711
                  tunnel: [w739] -> w714
                  tunnel: [w738] -> w717
                  tunnel: w712 -> [w738]
                  tunnel: w711 -> [w739]
                  frame #0 {
                    w732 = u16 1 items=["Get&Set", "Get", "Set"] ("Mode")
                    n232 = call "ColorTemp.vi"("DeviceNo"=w730, "Mode"=w732, "ChildNo"=w729, "Error_In"=w727) -> ("Error?"=w731:bool, "GetColor"=w722:cluster{"Mode":u32, "R":u32, "G":u32, "B":u32}, "Error_Out"=w728:T6)  [unwired: 1 in, 8 out]
                    n233 = Unbundle By Name(w722) -> ("Mode"=w721:u32, "R"=w720:u32, "G"=w719:u32, "B"=w718:u32)
                    n234 = case shown="1..6" w721 {
                      tunnel: [_ w737] -> w726
                      tunnel: [_ w736] -> w725
                      tunnel: [_ w735] -> w724
                      tunnel: w720 -> [_ w737]
                      tunnel: w719 -> [_ w736]
                      tunnel: w718 -> [_ w735]
                      frame Default {
                      }
                      frame 1..6 {
                      }
                    }
                    n235 = case shown="3..6" w721 {
                      tunnel: [FALSE ("表示") TRUE ("表示")] -> w723
                      frame 3..6 {
                      }
                      frame 1, 2, Default {
                      }
                    }
                    n236 = property on="Red" class="Slide (strict)"("Value"=w726) -> ()  [unwired: 2 in, 2 out]
                    n237 = property on="Green" class="Slide (strict)"("Value"=w725) -> ()  [unwired: 2 in, 2 out]
                    n238 = property on="Blue" class="Slide (strict)"("Value"=w724) -> ()  [unwired: 2 in, 2 out]
                    n239 = property on="Color_Cover" class="Str"("Visible"=w723) -> ()  [unwired: 2 in, 2 out]
                  }
                  frame #1 {
                    n240 = case shown="False" w738 {
                      frame False {
                        n241 = global write "global.vi" "OptionOK"(TRUE ("OptionOK")) -> ()
                      }
                      frame True {
                      }
                    }
                  }
                }
              }
              frame True {
              }
            }
          }
          event "Color-Temp.Red": Value Change {
            w751 = u16 2 items=["Get&Set", "Get", "Set"] ("Mode")
            n242 = event-data() -> ("NewVal"=w743:u32)  [unwired: 1 out]
            n243 = property on="Green" class="Slide (strict)"() -> ("Value"=w747:u32)  [unwired: 2 in, 2 out]
            n244 = property on="Blue" class="Slide (strict)"() -> ("Value"=w746:u32)  [unwired: 2 in, 2 out]
            n245 = property on="Mode" class="Ring (strict)"() -> ("Value"=w744:u32)  [unwired: 2 in, 2 out]
            n246 = Bundle("Value"=w744, "NewVal"=w743, "Value"=w747, "Value"=w746) -> (w745:T11)  [unwired: 1 out]
            n247 = call "ColorTemp.vi"("DeviceNo"=w753, "Mode"=w751, "ChildNo"=w752, "Error_In"=w748, "SetColor"=w745) -> ("Error?"=w750:bool, "Error_Out"=w749:T6)  [unwired: 9 out]
            n248 = case shown="False" w750 {
              tunnel: w749 -> [w759 w787]
              tunnel: w753 -> [w762 _]
              tunnel: w752 -> [w761 _]
              tunnel: [w763 TRUE ("Error?")] -> w755
              tunnel: [w760 w787] -> w754
              frame False {
                n249 = flat-sequence {
                  tunnel: w762 -> [w776]
                  tunnel: w761 -> [w775]
                  tunnel: w759 -> [w773]
                  tunnel: [w777] -> w758
                  tunnel: [w774] -> w757
                  tunnel: [w785] -> w760
                  tunnel: [w784] -> w763
                  tunnel: w758 -> [w784]
                  tunnel: w757 -> [w785]
                  frame #0 {
                    w778 = u16 1 items=["Get&Set", "Get", "Set"] ("Mode")
                    n250 = call "ColorTemp.vi"("DeviceNo"=w776, "Mode"=w778, "ChildNo"=w775, "Error_In"=w773) -> ("Error?"=w777:bool, "GetColor"=w768:cluster{"Mode":u32, "R":u32, "G":u32, "B":u32}, "Error_Out"=w774:T6)  [unwired: 1 in, 8 out]
                    n251 = Unbundle By Name(w768) -> ("Mode"=w767:u32, "R"=w766:u32, "G"=w765:u32, "B"=w764:u32)
                    n252 = case shown="1..6" w767 {
                      tunnel: [_ w783] -> w772
                      tunnel: [_ w782] -> w771
                      tunnel: [_ w781] -> w770
                      tunnel: w766 -> [_ w783]
                      tunnel: w765 -> [_ w782]
                      tunnel: w764 -> [_ w781]
                      frame Default {
                      }
                      frame 1..6 {
                      }
                    }
                    n253 = case shown="3..6" w767 {
                      tunnel: [FALSE ("表示") TRUE ("表示")] -> w769
                      frame 3..6 {
                      }
                      frame 1, 2, Default {
                      }
                    }
                    n254 = property on="Red" class="Slide (strict)"("Value"=w772) -> ()  [unwired: 2 in, 2 out]
                    n255 = property on="Green" class="Slide (strict)"("Value"=w771) -> ()  [unwired: 2 in, 2 out]
                    n256 = property on="Blue" class="Slide (strict)"("Value"=w770) -> ()  [unwired: 2 in, 2 out]
                    n257 = property on="Color_Cover" class="Str"("Visible"=w769) -> ()  [unwired: 2 in, 2 out]
                  }
                  frame #1 {
                    n258 = case shown="False" w784 {
                      frame False {
                        n259 = global write "global.vi" "OptionOK"(TRUE ("OptionOK")) -> ()
                      }
                      frame True {
                      }
                    }
                  }
                }
              }
              frame True {
              }
            }
          }
          event "Color-Temp.Green": Value Change {
            w797 = u16 2 items=["Get&Set", "Get", "Set"] ("Mode")
            n260 = event-data() -> ("NewVal"=w790:u32)  [unwired: 1 out]
            n261 = property on="Blue" class="Slide (strict)"() -> ("Value"=w793:u32)  [unwired: 2 in, 2 out]
            n262 = property on="Mode" class="Ring (strict)"() -> ("Value"=w791:u32)  [unwired: 2 in, 2 out]
            n263 = property on="Red" class="Slide (strict)"() -> ("Value"=w789:u32)  [unwired: 2 in, 2 out]
            n264 = Bundle("Value"=w791, "Value"=w789, "NewVal"=w790, "Value"=w793) -> (w792:T12)  [unwired: 1 out]
            n265 = call "ColorTemp.vi"("DeviceNo"=w799, "Mode"=w797, "ChildNo"=w798, "Error_In"=w794, "SetColor"=w792) -> ("Error?"=w796:bool, "Error_Out"=w795:T6)  [unwired: 9 out]
            n266 = case shown="False" w796 {
              tunnel: w795 -> [w805 w833]
              tunnel: w799 -> [w808 _]
              tunnel: w798 -> [w807 _]
              tunnel: [w809 TRUE ("Error?")] -> w801
              tunnel: [w806 w833] -> w800
              frame False {
                n267 = flat-sequence {
                  tunnel: w808 -> [w822]
                  tunnel: w807 -> [w821]
                  tunnel: w805 -> [w819]
                  tunnel: [w823] -> w804
                  tunnel: [w820] -> w803
                  tunnel: [w831] -> w806
                  tunnel: [w830] -> w809
                  tunnel: w804 -> [w830]
                  tunnel: w803 -> [w831]
                  frame #0 {
                    w824 = u16 1 items=["Get&Set", "Get", "Set"] ("Mode")
                    n268 = call "ColorTemp.vi"("DeviceNo"=w822, "Mode"=w824, "ChildNo"=w821, "Error_In"=w819) -> ("Error?"=w823:bool, "GetColor"=w814:cluster{"Mode":u32, "R":u32, "G":u32, "B":u32}, "Error_Out"=w820:T6)  [unwired: 1 in, 8 out]
                    n269 = Unbundle By Name(w814) -> ("Mode"=w813:u32, "R"=w812:u32, "G"=w811:u32, "B"=w810:u32)
                    n270 = case shown="1..6" w813 {
                      tunnel: [_ w829] -> w818
                      tunnel: [_ w828] -> w817
                      tunnel: [_ w827] -> w816
                      tunnel: w812 -> [_ w829]
                      tunnel: w811 -> [_ w828]
                      tunnel: w810 -> [_ w827]
                      frame Default {
                      }
                      frame 1..6 {
                      }
                    }
                    n271 = case shown="3..6" w813 {
                      tunnel: [FALSE ("表示") TRUE ("表示")] -> w815
                      frame 3..6 {
                      }
                      frame 1, 2, Default {
                      }
                    }
                    n272 = property on="Red" class="Slide (strict)"("Value"=w818) -> ()  [unwired: 2 in, 2 out]
                    n273 = property on="Green" class="Slide (strict)"("Value"=w817) -> ()  [unwired: 2 in, 2 out]
                    n274 = property on="Blue" class="Slide (strict)"("Value"=w816) -> ()  [unwired: 2 in, 2 out]
                    n275 = property on="Color_Cover" class="Str"("Visible"=w815) -> ()  [unwired: 2 in, 2 out]
                  }
                  frame #1 {
                    n276 = case shown="False" w830 {
                      frame False {
                        n277 = global write "global.vi" "OptionOK"(TRUE ("OptionOK")) -> ()
                      }
                      frame True {
                      }
                    }
                  }
                }
              }
              frame True {
              }
            }
          }
          event "Color-Temp.Blue": Value Change {
            w843 = u16 2 items=["Get&Set", "Get", "Set"] ("Mode")
            n278 = event-data() -> ("NewVal"=w836:u32)  [unwired: 1 out]
            n279 = property on="Mode" class="Ring (strict)"() -> ("Value"=w837:u32)  [unwired: 2 in, 2 out]
            n280 = property on="Red" class="Slide (strict)"() -> ("Value"=w835:u32)  [unwired: 2 in, 2 out]
            n281 = property on="Green" class="Slide (strict)"() -> ("Value"=w839:u32)  [unwired: 2 in, 2 out]
            n282 = Bundle("Value"=w837, "Value"=w835, "Value"=w839, "NewVal"=w836) -> (w838:T13)  [unwired: 1 out]
            n283 = call "ColorTemp.vi"("DeviceNo"=w845, "Mode"=w843, "ChildNo"=w844, "Error_In"=w840, "SetColor"=w838) -> ("Error?"=w842:bool, "Error_Out"=w841:T6)  [unwired: 9 out]
            n284 = case shown="False" w842 {
              tunnel: w841 -> [w851 w879]
              tunnel: w845 -> [w854 _]
              tunnel: w844 -> [w853 _]
              tunnel: [w855 TRUE ("Error?")] -> w847
              tunnel: [w852 w879] -> w846
              frame False {
                n285 = flat-sequence {
                  tunnel: w854 -> [w868]
                  tunnel: w853 -> [w867]
                  tunnel: w851 -> [w865]
                  tunnel: [w869] -> w850
                  tunnel: [w866] -> w849
                  tunnel: [w877] -> w852
                  tunnel: [w876] -> w855
                  tunnel: w850 -> [w876]
                  tunnel: w849 -> [w877]
                  frame #0 {
                    w870 = u16 1 items=["Get&Set", "Get", "Set"] ("Mode")
                    n286 = call "ColorTemp.vi"("DeviceNo"=w868, "Mode"=w870, "ChildNo"=w867, "Error_In"=w865) -> ("Error?"=w869:bool, "GetColor"=w860:cluster{"Mode":u32, "R":u32, "G":u32, "B":u32}, "Error_Out"=w866:T6)  [unwired: 1 in, 8 out]
                    n287 = Unbundle By Name(w860) -> ("Mode"=w859:u32, "R"=w858:u32, "G"=w857:u32, "B"=w856:u32)
                    n288 = case shown="1..6" w859 {
                      tunnel: [_ w875] -> w864
                      tunnel: [_ w874] -> w863
                      tunnel: [_ w873] -> w862
                      tunnel: w858 -> [_ w875]
                      tunnel: w857 -> [_ w874]
                      tunnel: w856 -> [_ w873]
                      frame Default {
                      }
                      frame 1..6 {
                      }
                    }
                    n289 = case shown="3..6" w859 {
                      tunnel: [FALSE ("表示") TRUE ("表示")] -> w861
                      frame 3..6 {
                      }
                      frame 1, 2, Default {
                      }
                    }
                    n290 = property on="Red" class="Slide (strict)"("Value"=w864) -> ()  [unwired: 2 in, 2 out]
                    n291 = property on="Green" class="Slide (strict)"("Value"=w863) -> ()  [unwired: 2 in, 2 out]
                    n292 = property on="Blue" class="Slide (strict)"("Value"=w862) -> ()  [unwired: 2 in, 2 out]
                    n293 = property on="Color_Cover" class="Str"("Visible"=w861) -> ()  [unwired: 2 in, 2 out]
                  }
                  frame #1 {
                    n294 = case shown="False" w876 {
                      frame False {
                        n295 = global write "global.vi" "OptionOK"(TRUE ("OptionOK")) -> ()
                      }
                      frame True {
                      }
                    }
                  }
                }
              }
              frame True {
              }
            }
          }
          event "BitSelect.BitShift": Value Change {
            n296 = event-data() -> ("NewVal"=w887:dbl)  [unwired: 1 out]
            n297 = To Unsigned Word Integer(number=w887) -> (unsigned 16bit integer=w886:u16)
            n298 = flat-sequence {
              tunnel: w890 -> [w899]
              tunnel: w886 -> [w895]
              tunnel: w885 -> [w894]
              tunnel: w884 -> [w893]
              tunnel: [w898] -> w883
              tunnel: [w897] -> w882
              tunnel: w881 -> [w892]
              tunnel: [w900] -> w888
              tunnel: [w901] -> w889
              tunnel: w883 -> [w901]
              tunnel: w882 -> [w900]
              frame #0 {
                w896 = u16 2 items=["Get&Set", "Get", "Set"] ("Mode")
                n299 = call "TransferOption.vi"("Depth"=w892, "Mode"=w896, "Error_In"=w899, "Newn8BitSel"=w895, "ChildNo"=w894, "DeviceNo"=w893) -> ("Error_Out"=w898:T6, "Error?"=w897:bool)  [unwired: 3 out]
              }
              frame #1 {
                n300 = case shown="False" w900 {
                  frame False {
                    n301 = global write "global.vi" "OptionOK"(TRUE ("OptionOK")) -> ()
                  }
                  frame True {
                  }
                }
              }
            }
          }
          event "I/O PortSetting.ExternalOut1", "I/O PortSetting.ExternalOut2", "I/O PortSetting.ExternalOut3", "I/O PortSetting.ExternalOut4": Value Change {
            n302 = event-data() -> ()  [unwired: 7 out]
            n303 = flat-sequence {
              tunnel: w910 -> [w925]
              tunnel: w909 -> [w924]
              tunnel: w908 -> [w923]
              tunnel: [w922] -> w905
              tunnel: [w921] -> w904
              tunnel: [w936] -> w906
              tunnel: [w935] -> w907
              tunnel: w905 -> [w935]
              tunnel: w904 -> [w936]
              frame #0 {
                w934 = u16 2 items=["Get&Set", "Get", "Set"] ("Mode")
                n304 = property on="ExternalOut4" class="Ring (strict)"() -> ("Value"=w916:u16, "Visible"=w917:bool)  [unwired: 2 in, 2 out]
                n305 = property on="ExternalOut3" class="Ring (strict)"() -> ("Value"=w919:u16, "Visible"=w920:bool)  [unwired: 2 in, 2 out]
                n306 = property on="ExternalOut1" class="Ring (strict)"() -> ("Value"=w931:u16, "Visible"=w933:bool)  [unwired: 2 in, 2 out]
                n307 = property on="ExternalOut2" class="Ring (strict)"() -> ("Value"=w930:u16, "Visible"=w932:bool)  [unwired: 2 in, 2 out]
                n308 = Select(t=w916, s=w917, f=u16 0) -> (s? t:f=w911:u16)
                n309 = Select(t=w919, s=w920, f=u16 0) -> (s? t:f=w912:u16)
                n310 = Select(t=w931, s=w933, f=u16 0) -> (s? t:f=w914:u16)
                n311 = Select(t=w930, s=w932, f=u16 0) -> (s? t:f=w913:u16)
                n312 = Build Array(w914, w913, w912, w911) -> (w927:u16[])
                n313 = To Unsigned Long Integer(number=w927) -> (unsigned 32bit integer=w926:u32[])
                n314 = call "ExternalOUT.vi"("nDeviceNo"=w924, "Mode"=w934, "nChildNo"=w923, "NewExternalOutMode"=w926, "Error_In"=w925) -> ("Error?"=w922:bool, "Error_Out"=w921:T7)  [unwired: 9 out]
              }
              frame #1 {
                n315 = case shown="False" w935 {
                  frame False {
                    n316 = global write "global.vi" "OptionOK"(TRUE ("OptionOK")) -> ()
                  }
                  frame True {
                  }
                }
              }
            }
          }
          event "I/O PortSetting.ExternalIn1", "I/O PortSetting.ExternalIn2", "I/O PortSetting.ExternalIn3": Value Change {
            n317 = event-data() -> ()  [unwired: 7 out]
            n318 = flat-sequence {
              tunnel: w945 -> [w955]
              tunnel: w944 -> [w954]
              tunnel: w943 -> [w953]
              tunnel: [w951] -> w940
              tunnel: [w950] -> w939
              tunnel: [w966] -> w941
              tunnel: [w967] -> w942
              tunnel: w940 -> [w967]
              tunnel: w939 -> [w966]
              frame #0 {
                w952 = u16 2 items=["Get&Set", "Get", "Set"] ("Mode")
                n319 = property on="ExternalIn3" class="Ring (strict)"() -> ("Value"=w948:u16, "Visible"=w947:bool)  [unwired: 2 in, 2 out]
                n320 = property on="ExternalIn1" class="Ring (strict)"() -> ("Value"=w959:u16, "Visible"=w958:bool)  [unwired: 2 in, 2 out]
                n321 = property on="ExternalIn2" class="Ring (strict)"() -> ("Value"=w957:u16, "Visible"=w956:bool)  [unwired: 2 in, 2 out]
                n322 = Select(t=w948, s=w947, f=u16 0) -> (s? t:f=w946:u16)
                n323 = Select(t=w957, s=w956, f=u16 0) -> (s? t:f=w964:u16)
                n324 = Select(t=w959, s=w958, f=u16 0) -> (s? t:f=w963:u16)
                n325 = Build Array(w963, w964, w946) -> (w965:u16[])
                n326 = To Unsigned Long Integer(number=w965) -> (unsigned 32bit integer=w960:u32[])
                n327 = call "ExternalIN.vi"("nDeviceNo"=w954, "Mode"=w952, "nChildNo"=w953, "NewExternalInMode"=w960, "Error_In"=w955) -> ("Error?"=w950:bool, "Error_Out"=w951:T7)  [unwired: 9 out]
              }
              frame #1 {
                n328 = case shown="False" w966 {
                  frame False {
                    n329 = global write "global.vi" "OptionOK"(TRUE ("OptionOK")) -> ()
                  }
                  frame True {
                  }
                }
              }
            }
          }
          event "PartitionNo", "Equalize": Value Change {
            # "PartitionCheck"
            n330 = event-data() -> ("CtlRef"=w974:refnum<vi>)  [unwired: 6 out]
            n331 = control-ref of="Equalize"() -> (w973:refnum<vi>)
            n332 = Unbundle By Name(w1000) -> ("error"=w1004:errorcluster)
            n333 = Equal?(x=w974, y=w973) -> (x = y?=w972:bool)
            n334 = call "PDC_GetMaxPartition.vi"("error in (no error)"=w1004, "ChildNo"=w986, "DeviceNo"=w987) -> ("error out"=w1001:errorcluster, "Block"=w982:u32, "Count"=w983:u32, "ReturnValue"=w1002:u32, "ErrorCode"=w1003:u32)  [unwired: 4 out]
            n335 = call "Error.vi"("error in (no error)"=w1001, "ErrorCode"=w1003, "ReturnValue"=w1002) -> ("Error_Out"=w999:T6, "Error?"=w980:bool)  [unwired: 7 out]
            n336 = case shown="False" w980 {
              tunnel: w999 -> [w1031 w1032]
              tunnel: w987 -> [w1023 w1035]
              tunnel: w986 -> [w1022 w1034]
              tunnel: [w1028 w1032] -> w985
              tunnel: [w1025 _] -> w984
              tunnel: [w1024 _] -> w981
              tunnel: [w1023 w1035] -> w979
              tunnel: [w1022 w1034] -> w978
              tunnel: [w1021 TRUE ("Error?")] -> w975
              frame False {
                n337 = Unbundle By Name(w1031) -> ("error"=w1030:errorcluster)
                n338 = call "PDC_GetPartitionList.vi"("DeviceNo"=w1023, "ChildNo"=w1022, "error in (no error)"=w1030) -> ("ReturnValue"=w1027:u32, "Count"=w1025:u32, "Blocks"=w1024:u32[], "ErrorCode"=w1026:u32, "error out"=w1029:errorcluster)  [unwired: 8 out]
                n339 = call "Error.vi"("error in (no error)"=w1029, "ErrorCode"=w1026, "ReturnValue"=w1027) -> ("Error_Out"=w1028:T6, "Error?"=w1021:bool)  [unwired: 7 out]
              }
              frame True {
                # "Error"
              }
            }
            n340 = property on="PartitionNo" class="DigNum (strict)"() -> ("Value"=w970:u32)  [unwired: 2 in, 2 out]
            n341 = local read "PartitionList"() -> (w969:T4)
            n342 = call "SetpBlock.vi"("PartitionList"=w969, "Blocks"=w981, "PBlock"=w982, "PCount"=w983, "NewPartitionNo"=w970, "NowPartitionNo"=w984) -> ("Block"=w998:i32[])  [unwired: 5 out]
            n343 = case shown="False" w975 {
              tunnel: w998 -> [w1013 _]
              tunnel: [w1012 w1018] -> w997
              tunnel: [w1011 TRUE ("Error?")] -> w990
              tunnel: w985 -> [w1010 w1018]
              tunnel: w970 -> [w1008 _]
              tunnel: w979 -> [w1007 w1020]
              tunnel: w978 -> [w1006 w1019]
              tunnel: [w1007 w1020] -> w977
              tunnel: [w1006 w1019] -> w976
              frame False {
                n344 = Unbundle By Name(w1010) -> ("error"=w1009:errorcluster)
                n345 = call "PDC_SetPartitionList.vi"("Blocks"=w1013, "error in (no error)"=w1009, "Count"=w1008, "ChildNo"=w1006, "DeviceNo"=w1007) -> ("error out"=w1016:errorcluster, "ReturnValue"=w1015:u32, "ErrorCode"=w1014:u32)  [unwired: 4 out]
                n346 = call "Error.vi"("error in (no error)"=w1016, "ErrorCode"=w1014, "ReturnValue"=w1015) -> ("Error_Out"=w1012:T6, "Error?"=w1011:bool)  [unwired: 7 out]
              }
              frame True {
                # "Error"
              }
            }
            n347 = Not Equal?(x=w983, y=u32 1) -> (x != y?=w988:bool)
            n348 = case shown="False" w990 {
              selector: w990 -> [w1047 _]
              tunnel: w997 -> [w1050 w1083]
              tunnel: [w1040 w1083] -> w995
              tunnel: [w1042 TRUE ("Error?")] -> w996
              tunnel: w977 -> [w1049 _]
              tunnel: w976 -> [w1048 _]
              tunnel: [w1046 u32 0 ("pCount")] -> w991
              tunnel: [w1045 _] -> w992
              tunnel: [w1044 _] -> w993
              tunnel: [w1037 u32 1 ("pNo")] -> w994
              tunnel: w988 -> [w1036 _]
              frame False {
                n349 = case shown="True" w1036 {
                  tunnel: w1049 -> [w1065 w1070]
                  tunnel: w1048 -> [w1064 w1069]
                  tunnel: w1050 -> [w1068 w1080]
                  tunnel: [w1068 w1075] -> w1041
                  tunnel: [w1067 w1074] -> w1043
                  tunnel: w1047 -> [w1067 _]
                  tunnel: [u32 1 ("pCount") w1073] -> w1046
                  tunnel: [_ w1072] -> w1045
                  tunnel: [_ w1071] -> w1044
                  tunnel: [w1065 w1070] -> w1039
                  tunnel: [w1064 w1069] -> w1038
                  frame False {
                    # "Not Support"
                  }
                  frame True {
                    n350 = Unbundle By Name(w1080) -> ("error"=w1079:errorcluster)
                    n351 = call "PDC_GetPartitionList.vi"("DeviceNo"=w1070, "ChildNo"=w1069, "error in (no error)"=w1079) -> ("ReturnValue"=w1077:u32, "Count"=w1073:u32, "Frames"=w1072:u32[], "Blocks"=w1071:u32[], "ErrorCode"=w1076:u32, "error out"=w1078:errorcluster)  [unwired: 7 out]
                    n352 = call "Error.vi"("error in (no error)"=w1078, "ErrorCode"=w1076, "ReturnValue"=w1077) -> ("Error_Out"=w1075:T6, "Error?"=w1074:bool)  [unwired: 7 out]
                    n353 = property on="PartitionNo" class="DigNum (strict)"("Value"=w1073) -> ()  [unwired: 2 in, 2 out]
                  }
                }
                n354 = case shown="False" w1043 {
                  tunnel: [w1055 TRUE] -> w1042
                  tunnel: w1041 -> [w1060 w1063]
                  tunnel: [w1056 w1063] -> w1040
                  tunnel: w1039 -> [w1053 _]
                  tunnel: w1038 -> [w1052 _]
                  tunnel: [w1051 u32 1 ("pNo")] -> w1037
                  frame False {
                    n355 = Unbundle By Name(w1060) -> ("error"=w1059:errorcluster)
                    n356 = call "PDC_GetCurrentPartition.vi"("error in (no error)"=w1059, "ChildNo"=w1052, "DeviceNo"=w1053) -> ("error out"=w1057:errorcluster, "No"=w1051:u32, "ReturnValue"=w1058:u32, "ErrorCode"=w1054:u32)  [unwired: 5 out]
                    n357 = call "Error.vi"("error in (no error)"=w1057, "ErrorCode"=w1054, "ReturnValue"=w1058) -> ("Error_Out"=w1056:T6, "Error?"=w1055:bool)  [unwired: 7 out]
                  }
                  frame True {
                    # "Error"
                  }
                }
              }
              frame True {
                # "Error"
              }
            }
            n358 = stacked-sequence {
              seq-local: [w1091 _] -> [_ w1129]
              tunnel: w982 -> [w1090 _]
              tunnel: w983 -> [w1095 _]
              tunnel: w991 -> [w1093 w1134]
              tunnel: w992 -> [w1088 w1133]
              tunnel: w993 -> [w1089 w1132]
              tunnel: w994 -> [_ w1128]
              tunnel: w970 -> [w1086 _]
              tunnel: w969 -> [w1085 _]
              frame #0 {
                n359 = Equal To 0?(x=w1090) -> (x = 0?=w1091:bool)
                n360 = Less Or Equal?(x=w1095, y=u32 8) -> (x <= y?=w1098:bool)
                n361 = Select(t=u8 2 ("無効"), s=w1091, f=u8 0 ("無効")) -> (s? t:f=w1100:u8)
                n362 = property on="Block" class="DigNum (strict)"("Disabled"=w1100) -> ()  [unwired: 2 in, 2 out]
                n363 = case shown="False" w1098 {
                  tunnel: [w1122 w1126] -> w1097
                  tunnel: [w1124 FALSE] -> w1096
                  tunnel: w1093 -> [w1121 w1126]
                  frame False {
                    n364 = Greater?(x=w1121, y=u32 8 ("pCount")) -> (0:w1124:bool)
                    n365 = Select(t=u32 8 ("pCount"), s=w1124, f=w1121) -> (s? t:f=w1122:u32)
                  }
                  frame True {
                  }
                }
                n366 = case shown="False" w1091 {
                  tunnel: [w1115 ""] -> w1092
                  tunnel: w1090 -> [w1105 _]
                  tunnel: w1089 -> [w1103 _]
                  tunnel: w1088 -> [w1104 _]
                  tunnel: [TRUE FALSE] -> w1087
                  tunnel: w1086 -> [_ _]
                  tunnel: w1085 -> [_ _]
                  frame False {
                    n367 = Add Array Elements(numeric array=w1104) -> (sum=w1109:u32)
                    n368 = Add Array Elements(numeric array=w1103) -> (sum=w1108:u32)
                    n369 = Divide(x=w1109, y=w1108) -> (x/y=w1107:dbl)
                    n370 = Number To Decimal String(number=w1108) -> (decimal integer string=w1113:string)  [unwired: 1 out]
                    n371 = Number To Decimal String(number=w1105) -> (decimal integer string=w1110:string)  [unwired: 1 out]
                    n372 = Concatenate Strings(w1113, "/", w1110) -> (w1111:string)
                    n373 = Format Value(format string="(%d Frames/Block)" ("形式文字列"), value (0)=w1107) -> (output string=w1118:string)  [unwired: 1 out]
                    n374 = Concatenate Strings("Used blocks : " ("形式文字列"), w1111, "\r\n", w1118) -> (w1115:string)
                  }
                  frame True {
                  }
                }
                n375 = property on="PartitionList" class="Arr (strict)"("Number of Rows"=w1097, "VertScroll"=w1096) -> ()  [unwired: 2 in, 2 out]
                n376 = property on="Frame" class="Slide (strict)"("Scale.Minimum"=0.0 ("データエントリ制限:最小"), "Scale.Maximum"=w1093) -> ()  [unwired: 2 in, 2 out]
                n377 = local write "BlockInfo"(w1092) -> ()
                n378 = property on="Equalize" class="Bool"("Visible"=w1087) -> ()  [unwired: 2 in, 2 out]
              }
              frame #1 {
                # "<-CurrentPartition"
                n379 = for {
                  N: w1134 -> [_]
                  tunnel: w1133 -> [w1153]
                  tunnel: w1132 -> [w1152]
                  shift-right: [w1154] -> w1130
                  shift-left: T4 [{"Check"=TRUE, "No"="", "Frame"=0, "FrameNo"="", "Block"=0}, {"Check"=FALSE, "No"="", "Frame"=0, "FrameNo"="", "Block"=0}, {"Check"=FALSE, "No"="", "Frame"=0, "FrameNo"="", "Block"=0}, {"Check"=FALSE, "No"="", "Frame"=0, "FrameNo"="", "Block"=0}, {"Check"=FALSE, "No"="", "Frame"=0, "FrameNo"="", "Block"=0}, {"Check"=FALSE, "No"="", "Frame"=0, "FrameNo"="", "Block"=0}, {"Check"=FALSE, "No"="", "Frame"=0, "FrameNo"="", "Block"=0}, {"Check"=FALSE, "No"="", "Frame"=0, "FrameNo"="", "Block"=0}, {"Check"=FALSE, "No"="", "Frame"=0, "FrameNo"="", "Block"=0}, {"Check"=FALSE, "No"="", "Frame"=0, "FrameNo"="", "Block"=0}, {"Check"=FALSE, "No"="", "Frame"=0, "FrameNo"="", "Block"=0}, {"Check"=FALSE, "No"="", "Frame"=0, "FrameNo"="", "Block"=0}, {"Check"=FALSE, "No"="", "Frame"=0, "FrameNo"="", "Block"=0}, {"Check"=FALSE, "No"="", "Frame"=0, "FrameNo"="", "Block"=0}, {"Check"=FALSE, "No"="", "Frame"=0, "FrameNo"="", "Block"=0}, {"Check"=FALSE, "No"="", "Frame"=0, "FrameNo"="", "Block"=0}, {"Check"=FALSE, "No"="", "Frame"=0, "FrameNo"="", "Block"=0}, {"Check"=FALSE, "No"="", "Frame"=0, "FrameNo"="", "Block"=0}, {"Check"=FALSE, "No"="", "Frame"=0, "FrameNo"="", "Block"=0}, {"Check"=FALSE, "No"="", "Frame"=0, "FrameNo"="", "Block"=0}, {"Check"=FALSE, "No"="", "Frame"=0, "FrameNo"="", "Block"=0}, {"Check"=FALSE, "No"="", "Frame"=0, "FrameNo"="", "Block"=0}, {"Check"=FALSE, "No"="", "Frame"=0, "FrameNo"="", "Block"=0}, {"Check"=FALSE, "No"="", "Frame"=0, "FrameNo"="", "Block"=0}, {"Check"=FALSE, "No"="", "Frame"=0, "FrameNo"="", "Block"=0}, {"Check"=FALSE, "No"="", "Frame"=0, "FrameNo"="", "Block"=0}, {"Check"=FALSE, "No"="", "Frame"=0, "FrameNo"="", "Block"=0}, {"Check"=FALSE, "No"="", "Frame"=0, "FrameNo"="", "Block"=0}, {"Check"=FALSE, "No"="", "Frame"=0, "FrameNo"="", "Block"=0}, {"Check"=FALSE, "No"="", "Frame"=0, "FrameNo"="", "Block"=0}, {"Check"=FALSE, "No"="", "Frame"=0, "FrameNo"="", "Block"=0}, {"Check"=FALSE, "No"="", "Frame"=0, "FrameNo"="", "Block"=0}, {"Check"=FALSE, "No"="", "Frame"=0, "FrameNo"="", "Block"=0}, {"Check"=FALSE, "No"="", "Frame"=0, "FrameNo"="", "Block"=0}, {"Check"=FALSE, "No"="", "Frame"=0, "FrameNo"="", "Block"=0}, {"Check"=FALSE, "No"="", "Frame"=0, "FrameNo"="", "Block"=0}, {"Check"=FALSE, "No"="", "Frame"=0, "FrameNo"="", "Block"=0}, {"Check"=FALSE, "No"="", "Frame"=0, "FrameNo"="", "Block"=0}, {"Check"=FALSE, "No"="", "Frame"=0, "FrameNo"="", "Block"=0}, {"Check"=FALSE, "No"="", "Frame"=0, "FrameNo"="", "Block"=0}, {"Check"=FALSE, "No"="", "Frame"=0, "FrameNo"="", "Block"=0}, {"Check"=FALSE, "No"="", "Frame"=0, "FrameNo"="", "Block"=0}, {"Check"=FALSE, "No"="", "Frame"=0, "FrameNo"="", "Block"=0}, {"Check"=FALSE, "No"="", "Frame"=0, "FrameNo"="", "Block"=0}, {"Check"=FALSE, "No"="", "Frame"=0, "FrameNo"="", "Block"=0}, {"Check"=FALSE, "No"="", "Frame"=0, "FrameNo"="", "Block"=0}, {"Check"=FALSE, "No"="", "Frame"=0, "FrameNo"="", "Block"=0}, {"Check"=FALSE, "No"="", "Frame"=0, "FrameNo"="", "Block"=0}, {"Check"=FALSE, "No"="", "Frame"=0, "FrameNo"="", "Block"=0}, {"Check"=FALSE, "No"="", "Frame"=0, "FrameNo"="", "Block"=0}, {"Check"=FALSE, "No"="", "Frame"=0, "FrameNo"="", "Block"=0}, {"Check"=FALSE, "No"="", "Frame"=0, "FrameNo"="", "Block"=0}, {"Check"=FALSE, "No"="", "Frame"=0, "FrameNo"="", "Block"=0}, {"Check"=FALSE, "No"="", "Frame"=0, "FrameNo"="", "Block"=0}, {"Check"=FALSE, "No"="", "Frame"=0, "FrameNo"="", "Block"=0}, {"Check"=FALSE, "No"="", "Frame"=0, "FrameNo"="", "Block"=0}, {"Check"=FALSE, "No"="", "Frame"=0, "FrameNo"="", "Block"=0}, {"Check"=FALSE, "No"="", "Frame"=0, "FrameNo"="", "Block"=0}, {"Check"=FALSE, "No"="", "Frame"=0, "FrameNo"="", "Block"=0}, {"Check"=FALSE, "No"="", "Frame"=0, "FrameNo"="", "Block"=0}, {"Check"=FALSE, "No"="", "Frame"=0, "FrameNo"="", "Block"=0}, {"Check"=FALSE, "No"="", "Frame"=0, "FrameNo"="", "Block"=0}, {"Check"=FALSE, "No"="", "Frame"=0, "FrameNo"="", "Block"=0}, {"Check"=FALSE, "No"="", "Frame"=0, "FrameNo"="", "Block"=0}] ("PartitionList") -> [w1151]
                  tunnel: w1129 -> [w1142]
                  tunnel: w1128 -> [w1137]
                  i -> [w1138]
                  n380 = Increment(x=w1138) -> (x+1=w1149:i32)
                  n381 = Increment(x=w1138) -> (x+1=w1136:i32)
                  n382 = Index Array(array=w1153, index=w1138) -> (element=w1145:u32)
                  n383 = Index Array(array=w1152, index=w1138) -> (element=w1141:u32)
                  n384 = Equal?(x=w1136, y=w1137) -> (x = y?=w1135:bool)
                  n385 = Format Value(format string="%03d" ("形式文字列"), value (0)=w1149) -> (output string=w1147:string)  [unwired: 1 out]
                  n386 = Index Array(array=w1151, index=w1138) -> (element=w1150:T8)
                  n387 = Select(t=u32 1, s=w1142, f=w1141) -> (s? t:f=w1139:u32)
                  n388 = Format Value(format string="%dFrame" ("形式文字列"), value (0)=w1145) -> (output string=w1144:string)  [unwired: 1 out]
                  n389 = Bundle By Name(cluster=w1150, "No"=w1147, "FrameNo"=w1144, "Block"=w1139, "Frame"=w1139, "Check"=w1135) -> (w1143:T8)
                  n390 = Replace Array Subset(array=w1151, new element=w1143, index=w1138) -> (w1154:T4)
                }
                n391 = local write "PartitionList"(w1130) -> ()
              }
            }
          }
          event "PartitionList": Value Change {
            n392 = event-data() -> ("OldVal"=w1165:T4, "NewVal"=w1164:T4)  [unwired: 5 out]
            n393 = for {
              tunnel: w1165 -> [w1277] mode=indexing
              tunnel: w1164 -> [w1276] mode=indexing
              tunnel: [w1275] -> w1163 mode=indexing
              tunnel: [w1274] -> w1162 mode=indexing
              n394 = Unbundle By Name(w1277) -> ("Check"=w1275:bool)
              n395 = Unbundle By Name(w1276) -> ("Check"=w1274:bool)
            }
            n396 = Not Equal?(x=w1163, y=w1162) -> (x != y?=w1161:bool)
            n397 = case shown="False" w1161 {
              tunnel: w1165 -> [w1176 w1262]
              tunnel: w1164 -> [w1167 w1261]
              tunnel: w1160 -> [w1179 w1259]
              tunnel: w1159 -> [_ _]
              tunnel: [w1172 w1256] -> w1158
              tunnel: [w1173 w1255] -> w1157
              tunnel: w1156 -> [w1170 w1254]
              tunnel: w1155 -> [w1169 w1253]
              frame False {
                # "Change Block"
                n398 = for {
                  tunnel: [w1247] -> w1171 mode=indexing
                  tunnel: w1167 -> [w1246] mode=indexing
                  n399 = Unbundle By Name(w1246) -> ("Block"=w1247:u32)
                }
                n400 = Unbundle By Name(w1179) -> ("error"=w1180:errorcluster)
                n401 = call "PDC_GetMaxPartition.vi"("error in (no error)"=w1180, "ChildNo"=w1169, "DeviceNo"=w1170) -> ("error out"=w1183:errorcluster, "Count"=w1168:u32, "ReturnValue"=w1182:u32, "ErrorCode"=w1181:u32)  [unwired: 5 out]
                n402 = call "Error.vi"("error in (no error)"=w1183, "ErrorCode"=w1181, "ReturnValue"=w1182) -> ("Error_Out"=w1175:T6, "Error?"=w1174:bool)  [unwired: 7 out]
                n403 = Add Array Elements(numeric array=w1171) -> (sum=w1178:u32)
                n404 = Greater Or Equal?(x=w1168, y=w1178) -> (x >= y?=w1177:bool)
                n405 = case shown="True" w1177 {
                  tunnel: w1176 -> [w1186 _]
                  tunnel: w1175 -> [w1184 w1195]
                  tunnel: w1174 -> [w1185 w1197]
                  tunnel: [w1185 w1196] -> w1173
                  tunnel: [w1184 w1194] -> w1172
                  tunnel: w1170 -> [_ w1193]
                  tunnel: w1169 -> [_ w1192]
                  tunnel: w1171 -> [_ w1191]
                  tunnel: w1170 -> [_ w1190]
                  tunnel: w1169 -> [_ w1189]
                  tunnel: w1168 -> [_ w1188]
                  tunnel: w1167 -> [_ w1187]
                  frame False {
                    # "MAX Over"
                    n406 = local write "PartitionList"(w1186) -> ()
                  }
                  frame True {
                    n407 = case shown="False" w1197 {
                      tunnel: [w1201 TRUE] -> w1196
                      tunnel: w1195 -> [w1214 w1244]
                      tunnel: [w1202 w1244] -> w1194
                      tunnel: w1193 -> [w1208 _]
                      tunnel: w1192 -> [w1207 _]
                      tunnel: w1191 -> [w1209 _]
                      tunnel: w1190 -> [w1204 _]
                      tunnel: w1189 -> [w1203 _]
                      tunnel: w1188 -> [w1200 _]
                      tunnel: w1187 -> [w1199 _]
                      frame False {
                        # "Block Update"
                        n408 = property on="PartitionNo" class="DigNum (strict)"() -> ("Value"=w1198:u32)  [unwired: 2 in, 2 out]
                        n409 = Unbundle By Name(w1214) -> ("error"=w1213:errorcluster)
                        n410 = call "PDC_SetPartitionList.vi"("Blocks"=w1209, "error in (no error)"=w1213, "Count"=w1198, "ChildNo"=w1207, "DeviceNo"=w1208) -> ("error out"=w1212:errorcluster, "ReturnValue"=w1211:u32, "ErrorCode"=w1210:u32)  [unwired: 4 out]
                        n411 = call "Error.vi"("error in (no error)"=w1212, "ErrorCode"=w1210, "ReturnValue"=w1211) -> ("Error_Out"=w1205:T6, "Error?"=w1206:bool)  [unwired: 7 out]
                        n412 = case shown="False" w1206 {
                          tunnel: w1205 -> [w1241 w1243]
                          tunnel: w1204 -> [w1239 _]
                          tunnel: w1203 -> [w1238 _]
                          tunnel: [w1234 w1243] -> w1202
                          tunnel: [w1233 TRUE ("Error?")] -> w1201
                          tunnel: w1200 -> [w1220 _]
                          tunnel: w1199 -> [w1218 _]
                          tunnel: w1198 -> [w1215 _]
                          frame False {
                            n413 = Unbundle By Name(w1241) -> ("error"=w1240:errorcluster)
                            n414 = Number To Decimal String(number=w1220) -> (decimal integer string=w1224:string)  [unwired: 1 out]
                            n415 = call "PDC_GetPartitionList.vi"("DeviceNo"=w1239, "ChildNo"=w1238, "error in (no error)"=w1240) -> ("ReturnValue"=w1237:u32, "Frames"=w1217:u32[], "Blocks"=w1216:u32[], "ErrorCode"=w1236:u32, "error out"=w1235:errorcluster)  [unwired: 8 out]
                            n416 = Add Array Elements(numeric array=w1217) -> (sum=w1223:u32)
                            n417 = Add Array Elements(numeric array=w1216) -> (sum=w1222:u32)
                            n418 = Divide(x=w1223, y=w1222) -> (x/y=w1221:dbl)
                            n419 = Number To Decimal String(number=w1222) -> (decimal integer string=w1227:string)  [unwired: 1 out]
                            n420 = Concatenate Strings(w1227, "/", w1224) -> (w1225:string)
                            n421 = Format Value(format string="(%d Frames/Block)" ("形式文字列"), value (0)=w1221) -> (output string=w1231:string)  [unwired: 1 out]
                            n422 = call "PartitionBlock.vi"("In_PartitionList"=w1218, "Blocks"=w1216, "Frames"=w1217, "Block"=w1215) -> ("Out_PartitionList"=w1219:T4)  [unwired: 7 out]
                            n423 = call "Error.vi"("error in (no error)"=w1235, "ErrorCode"=w1236, "ReturnValue"=w1237) -> ("Error_Out"=w1234:T6, "Error?"=w1233:bool)  [unwired: 7 out]
                            n424 = Concatenate Strings("Used blocks : " ("形式文字列"), w1225, "\r\n", w1231) -> (w1232:string)
                            n425 = local write "PartitionList"(w1219) -> ()
                            n426 = local write "BlockInfo"(w1232) -> ()
                          }
                          frame True {
                            # "Error"
                          }
                        }
                      }
                      frame True {
                        # "Error"
                      }
                    }
                  }
                }
              }
              frame True {
                # "Change CurrentPartition"
                n427 = Unbundle By Name(w1259) -> ("error"=w1258:errorcluster)
                n428 = for {
                  tunnel: w1262 -> [w1273] mode=indexing
                  tunnel: w1261 -> [w1272] mode=indexing
                  shift-right: [w1267] -> w1263
                  shift-left: w1261 -> [w1271]
                  tunnel: [w1264] -> w1252 mode=indexing
                  i -> [w1270]
                  n429 = Unbundle By Name(w1273) -> ("Check"=w1265:bool)
                  n430 = Unbundle By Name(w1272) -> ("Check"=w1266:bool)
                  n431 = Not Equal?(x=w1265, y=w1266) -> (x != y?=w1264:bool)
                  n432 = Index Array(array=w1271, index=w1270) -> (element=w1269:T8)
                  n433 = Bundle By Name(cluster=w1269, "Check"=w1264) -> (w1268:T8)
                  n434 = Replace Array Subset(array=w1271, new element=w1268, index=w1270) -> (w1267:T4)
                }
                n435 = local write "PartitionList"(w1263) -> ()
                n436 = Search 1D Array(1D array=w1252, element=TRUE ("要素")) -> (index of element=w1250:i32)  [unwired: 1 out]
                n437 = Increment(x=w1250) -> (x+1=w1249:i32)
                n438 = call "PDC_SetCurrentPartition.vi"("error in (no error)"=w1258, "No"=w1249, "ChildNo"=w1253, "DeviceNo"=w1254) -> ("error out"=w1257:errorcluster, "ReturnValue"=w1260:u32, "ErrorCode"=w1248:u32)  [unwired: 5 out]
                n439 = call "Error.vi"("error in (no error)"=w1257, "ErrorCode"=w1248, "ReturnValue"=w1260) -> ("Error_Out"=w1256:T6, "Error?"=w1255:bool)  [unwired: 7 out]
              }
            }
          }
        }
      }
    }
    frame #4 {
      n440 = Current VI's Path() -> (path=w1278:path)
      n441 = Strip Path(path=w1278) -> (name=w1279:string)  [unwired: 1 out]
      n442 = call <vilib>:"Close Panel.vi"("VI name"=w1279) -> ()  [unwired: 1 in, 10 out]
    }
  }
  n443 = property on="タブ制御器" class="TabCtl (strict)"("Value"=w1) -> ()  [unwired: 2 in, 2 out]
